vi "PH_Beamline_Chief.panel.vi"(0 "object ref":refnum<vi>, 5 "error in (no error)":errorcluster) -> (19 "error out":errorcluster)   [LabVIEW 2014, in "PH_Beamline_Chief.lvlib"]
doc: "By this VI a hardware switch can be monitored and switched. \n\nThe indicators \"FALSE\", \"TRUE\" and \"SWITCH STATE\" show the value of the Beckhoff-Tag: blue indicates bad tag status reference problems, darkgreen false and lightgreen true. If everything is working fine, \"FALSE\" and \"SWITCH STATE\" should show the same value, while \"TRUE\" has the opposite value. The caption of the sensors for \"FALSE\" and \"TRUE\" are taken out of the database. In case of only one or no sensor these GUI elements are not shown at all.\n\nThe oval button switches. It should be in the same state as the \"SWITCH STATE\" indicator. \n\n\"Delete Instance\" disconnects and removes the instance from the PCS.\n\n\nLicense Agreement for this software:\n\nCopyright (C)\nGesellschaft für Schwerionenforschung, GSI\nPlanckstr. 1\n64291 Darmstadt\nGermany\n\nContact: D.Beck@gsi.de \n\nThis program is free software; you can redistribute it and/or modify it under the terms of the GNU General Public License as published by the Free Software Foundation; either version 2 of the license, or (at your option) any later version.\n\nThis program is distributed in the hope that it will be useful, but WITHOUT ANYW ARRANTY; without even the implied warranty of MERCHANTABILITY or FITNESS FOR A PARTICULAR PURPOSE. See the GNU General License for more details (http://www.gnu.org).\n\nGesellschaft für Schwerionenforschung, GSI\nPlanckstr. 1, 64291 Darmstadt, Germany\nFor all questions and ideas contact: M.Richter@gsi.de, H.Brand@gsi.de or D.Beck@gsi.de.\nLast update: 18-DEC-2002"
uses:
  PH_Beamline_Chief.lvlib
  PH_Basics/PH_Common/Picture/PH_Picture.GUI Element 48x48.ctl
  PH_Basics/PH_Common/Picture/PH_Picture.GUI Element 36x36.ctl
  PH_Basics/PH_Common/Picture/PH_Picture.GUI Element 24x36.ctl
  PH_Basics/PH_Common/Picture/PH_Picture.GUI Element.ctl
  PH_Basics/PH_Common/Picture/PH_Picture.GUI Element 36x24.ctl
  PH_Basics/PH_Common/Picture/PH_Picture.GUI Element 60x12.ctl
  PH_Basics/PH_Common/Picture/PH_Picture.GUI Element 12x60.ctl
  PH_Beamline/PH_Beamline.Operation Mode.ctl
  PH_Beamline/PH_Beamline.Switch Instances.ctl
  PH_Beamline/PH_Beamline.6P Switch Instances.ctl
  PH_Beamline/PH_Beamline.Black Box Instances.ctl
  PH_Beamline/PH_Beamline.Switch GUI Instances.ctl
  PH_Beamline/PH_Beamline.Switch+6P Instances.ctl
  PH_Beamline_Chief.Settings.ctl
  PH_Beamline/PH_Beamline.Force Sensor Instances.ctl
  PH_Basics/PH_SystemInformation/PH_SystemInformation.GUI Refs.ctl
  PH_BL-Master/PH_BL-Master.GUI Refs.ctl
  PH_Beamline/PH_Beamline.GUI Refs.ctl
  CS_Core/CSObj/CSObj.lvlib
  PH_Basics/PH_Common/PH_Common.lvlib
  PH_BL-Master/PH_BL-Master.lvlib
  PH_Basics/PH_SystemInformation/PH_SystemInformation.lvlib
  PH_Basics/PH_Class/PH_Class.lvlib
  PH_Beamline/PH_Beamline.lvlib
  CS_Core/CSSystem/CSSystemLib/CSSystemLib.lvlib
panel:
  in  "Force Sensor Instances":T1="MM1_ForceSensor"
  in  "Switch and 6P Instances":T2="BL_Position_MM5::MA_MM5_6PGUI"
  in  "Switch GUI Instances":T3="Shutter_Exp_Laserbay_Interlock"
  in  "Black Box Instances":T4="PA_CH1_BB"
  in  "6P Switch Instances":T5="COS_Sensitivity_Switch"
  in  "Switch Instances":T6="MA01_CH1"
  out "Exp.-Shutters closed":bool
  in  "Remote Desktop Connection":bool
  out "PHELIX_Beckhoff_Watchdog":bool caption="Failure Beckhoff"
  out "PHELIX_Timing_Mode":enum32{"10 Hz", "0.5 Hz", "Shot"}(radio) caption="Modeselector"
  out "Emergency Off":u32(colorbox)
  out "Igni FR: Heating off":bool
  out "Igni MA 5: Heating off":bool
  out "Igni MA 4: Heating off":bool
  out "Igni MA 3: Heating off":bool
  out "Igni MA 2: Heating off":bool
  out "Igni MA 1: Heating off":bool
  in  "Z6 Main":bool
  in  "PCS Main":bool
  in  "PCS System Indicator":bool caption="PCS"
  in  "CoG":bool
  in  "Calibrator":bool
  in  "Image Statistician":bool
  out "Shutter_Exp3":bool=TRUE
  out "Shutter_Exp2":bool=TRUE
  out "Shutter_Exp1":bool=TRUE
  out "Shutter Exp 4 (Z6)":u32(colorbox)
  out "Shutter Exp 3":u32(colorbox)
  out "Shutter Exp 2":u32(colorbox)
  out "Shutter Exp 1":u32(colorbox)
  in  "Tab Control":T7(tab)=enum."In.-Box"
  in  "\"D:\\PCS\\Remote Access\\ns.rdp\"":bool caption="OK Button"
  out "ns Frontend ok":bool caption="ok"
  out "ns_WP_RR_6PWpGUI":T8
  in  "Hop 15":bool
  out "BL ns 8":u32(colorbox)
  out "NS_Shut_PA_BB":bool=TRUE
  out "BL ns 7":u32(colorbox)
  out "BL ns 6":u32(colorbox)
  out "BL ns 5":u32(colorbox)
  out "BL ns 4":u32(colorbox)
  out "BL ns 3":u32(colorbox)
  out "BL ns 2":u32(colorbox)
  out "BL ns 1":u32(colorbox)
  out "ns_Nearfield_Ring_Exit_ImageOperator":bool=TRUE
  out "ns_Nearfield_Ring_Exit_Cam":bool=TRUE
  out "ns_Farfield_Ring_Exit_ImageOperator":bool=TRUE
  out "ns_Farfield_Ring_Exit_Cam":bool=TRUE
  out "ns_Exit_Powermeter":bool=TRUE
  in  "Hop 23":bool
  in  "\"D:\\PCS\\Remote Access\\fs.rdp\"":bool caption="OK Button"
  out "fs Frontend ok":bool caption="ok"
  out "BL fs 17":u32(colorbox)
  out "BL fs 16":u32(colorbox)
  out "YLF_WP_6PWpGUI":T9
  out "fs_WP_Exit_6PWpGUI":T8
  out "fs_OO_Spectrometer":bool=TRUE
  out "BL fs 8":u32(colorbox)
  out "BL fs 10":u32(colorbox)
  out "fs_RR_Cavity_NF2GUI":T10
  out "fs_Stretcher_6PGUI":T10
  out "BL fs 15":u32(colorbox)
  out "FS_Shut_PA_BB":bool=TRUE
  out "BL fs 14":u32(colorbox)
  in  "Hop 3":bool
  out "BL fs 13":u32(colorbox)
  out "FS_Switch_YLF_BB":T10
  out "BL fs 12":u32(colorbox)
  out "BL fs 11":u32(colorbox)
  out "BL fs 7":u32(colorbox)
  out "BL fs 5":u32(colorbox)
  out "BL fs 9":u32(colorbox)
  out "BL fs 6":u32(colorbox)
  out "BL fs 4":u32(colorbox)
  out "BL fs 3":u32(colorbox)
  out "BL fs 2":u32(colorbox)
  out "BL fs 1":u32(colorbox)
  out "fs_Nearfield_Frontend_ImageOperator":bool=TRUE
  out "fs_Nearfield_Frontend_Cam":bool=TRUE caption="fs NF Exit Cam"
  out "fs_Synchrolock_Watch":bool=TRUE
  out "uOPA ok":bool caption="ok"
  in  "\"D:\\PCS\\Remote Access\\uOPA.rdp\"":bool caption="OK Button"
  out "BL uOPA 9":u32(colorbox)
  out "uOPA_Pump_OO_Spectrometer":bool=TRUE
  out "uOPA_Pump_WP_6PWpGUI":T8
  out "BL uOPA 8":u32(colorbox)=6618880
  out "BL uOPA 7":u32(colorbox)
  out "BL uOPA 6":u32(colorbox)
  out "BL uOPA 5":u32(colorbox)
  out "BL uOPA 4":u32(colorbox)
  out "BL uOPA 3":u32(colorbox)
  out "BL uOPA 2":u32(colorbox)
  out "BL uOPA 1":u32(colorbox)
  out "BL uOPA 0":u32(colorbox)
  in  "Hop 24":bool
  out "uOPA_Regen_Cam":bool=TRUE
  out "uOPA_Pump_Powermeter":bool=TRUE
  out "PA_Input_2_Beam_6PWpGUI":T8
  out "BL PA 21":u32(colorbox)
  out "BL PA 11":u32(colorbox)
  out "PA_ML_T3_Exit_6P4QGUI":T8 caption="PA Lens"
  out "PA_SA_6P4QGUI":T10
  out "PA_CH1_BB":T11 caption="CH"
  out "BL PA 4":u32(colorbox)
  out "PA_Input_Delay_6PGUI":T10
  out "BL PA 8":u32(colorbox)
  out "BL PA 7":u32(colorbox)
  out "BL PA 6":u32(colorbox)
  out "BL PA 5":u32(colorbox)
  out "BL PA 3":u32(colorbox)
  out "PA_non_delayed_BB":bool=TRUE
  out "PA_delayed_BB":bool=TRUE
  out "PA-Backreflection-Meas":bool=TRUE
  out "PA_PC_WP_2_BB":bool=TRUE
  in  "Hop 22":bool
  in  "Hop 16":bool
  out "BL PA 20":u32(colorbox)
  out "PA_PC_WP_BB":bool=TRUE
  out "PA_PiH_VSF2_6PGUI":T8
  out "BL PA 10":u32(colorbox)
  out "PA_Shut_Input_BB":bool=TRUE
  out "PA_PiH_VSF4_6PGUI":T8
  in  "Hop 6":bool
  in  "Hop 5":bool
  in  "Hop 4":bool
  out "PA_MM_P_Input_NF2GUI":T10
  out "PA_MM_C_Input_NF2GUI":T10
  out "BL PA 0":u32(colorbox)
  out "BL PA 16":u32(colorbox)
  out "BL PA 12":u32(colorbox)
  out "BL PA 14":u32(colorbox)
  out "PA_VacuumControl::PA_VacuumControl_Telescope 2":dbl=2000.0 caption="mbar" format="%#_2e"
  out "PA_VacuumControl::PA_VacuumControl_Telescope 3":dbl=2000.0 caption="mbar" format="%#_2e"
  out "PA_VacuumControl::PA_VacuumControl_Telescope 4":dbl=2000.0 caption="mbar" format="%#_2e"
  out "PA_VacuumControl::PA_VacuumControl_Bridge":dbl=2000.0 caption="mbar" format="%#_2e"
  out "BL PA 18":u32(colorbox)
  out "BL PA 17":u32(colorbox)
  out "PA_Bypass_Out":T10
  out "PA_Bypass_In":T10
  out "BL PA 22":u32(colorbox)
  out "PA_Switch_Lab_BB":T10
  out "PA_Exit_Shut_BB":bool=TRUE
  out "BL PA 19":u32(colorbox)
  out "BL PA 15":u32(colorbox)
  out "BL PA 13":u32(colorbox)
  out "PA_Nearfield_Input_ImageOperator":bool=TRUE
  out "PA_Nearfield_Input_Cam":bool=TRUE
  out "PA_Farfield_Input_ImageOperator":bool=TRUE
  out "PA_Farfield_Input_Cam":bool=TRUE
  out "BL PA 9":u32(colorbox)
  out "BL PA 1":u32(colorbox)
  out "PA_VacuumControl::PA_VacuumControl_Telescope 1":dbl=2000.0 caption="mbar" format="%#_2e"
  out "PA_VacuumControl::PA_VacuumControl_PA global":dbl=2000.0 caption="mbar" format="%#_2e"
  out "BL PA 2":u32(colorbox)
  out "PreAmp ok":bool caption="ok"
  in  "\"D:\\PCS\\Remote Access\\PA-Input.rdp\"":bool caption="OK Button"
  out "PA ED ok":bool caption="ok"
  in  "\"D:\\PCS\\Remote Access\\PA-Exit.rdp\"":bool caption="OK Button"
  out "PA_ED_FILT1_BB":bool=TRUE
  in  "Hop 7":bool
  out "PA_Exit_Powermeter":bool=TRUE
  out "BL PA ED 2":u32(colorbox)
  out "PA_WP_Exit_6PWpGUI":T9
  out "PA_Farfield_Exit_ImageOperator":bool=TRUE
  out "PA_Farfield_Exit_Cam":bool=TRUE caption="PA FF Exit Cam"
  out "PA_Nearfield_Exit_ImageOperator":bool=TRUE
  out "PA_Nearfield_Exit_Cam":bool=TRUE caption="PA NF Exit Cam"
  out "PA_ED_FILT2_BB":T9 caption="Filt 2"
  out "BL PA ED 1":u32(colorbox)
  out "MA_ML_In_6P4QGUI":T8 caption="PA Lens"
  out "PA_Bridge_CH_Input_MA_BB":T11 caption="CH"
  out "BL MA-IB 9":u32(colorbox)
  out "BL MA-IB 8":u32(colorbox)
  out "BL MA-IB 14":u32(colorbox)
  out "BL MA-IB 12":u32(colorbox)
  out "BL MA-IB 13":u32(colorbox)
  out "MA_Nearfield_PiH_out_ImageOperator":bool=TRUE
  out "MA_Nearfield_PiH_out_Cam":bool=TRUE
  out "MA_InB_IM_Out_Switch":T10
  out "MA_InB_DP_Out_Switch":bool=TRUE
  out "MA_InB_DP_In_Switch":bool=TRUE
  out "BL MA-IB 11":u32(colorbox)
  out "BL MA-IB 10":u32(colorbox)
  out "MA_InB_IM_In_Switch":T10
  out "BL MA-IB 7":u32(colorbox)
  out "BL MA-IB 6":u32(colorbox)
  out "BL MA-IB 5":u32(colorbox)
  out "MA_Diffusor_Inject_In_BB":bool=TRUE
  out "BL MA-IB 4":u32(colorbox)
  out "BL MA-IB 3":u32(colorbox)
  out "BL MA-IB 2":u32(colorbox)
  out "BL MA-IB 1":u32(colorbox)
  out "PA_C_MA_6PGUI":T10
  out "MA_Inject_In_ImageOperator":bool=TRUE
  out "MA_Inject_In_Cam":bool=TRUE
  out "MA_Inject_P_6PGUI":T10
  in  "Hop 2":bool
  in  "Hop 1":bool
  out "MA_Nearfield_PiH_in_ImageOperator":bool=TRUE
  out "MA_Nearfield_PiH_in_Cam":bool=TRUE
  out "MA_Inject_C_NF2GUI":T10
  out "MA_IB_Ready":bool
  out "PA_MA_Bridge_Input_Cam":bool=TRUE
  in  "\"D:\\PCS\\Remote Access\\MA.rdp\"":bool caption="OK Button"
  out "In.-Box ok":bool caption="ok"
  out "MM1_ForceSensor":bool
  in  "\"D:\\PCS\\Remote Access\\MA.rdp\" 2":bool caption="OK Button"
  out "FR+MT_Flowbox_off":bool caption="Flowboxes FR + MT off"
  out "MainAmp_Flowbox_off":bool caption="Flowboxes MA off"
  out "MainAmp ok":bool caption="ok"
  out "MA01_CH1":T11 caption="CH"
  out "MA01_CH2":T11 caption="CH"
  out "MA01_CH4":T11 caption="CH"
  out "MA01_CH3":T11 caption="CH"
  out "BL MA 3":u32(colorbox)
  out "BL MA 9":u32(colorbox)
  in  "Hop 11":bool
  out "BL MA 8":u32(colorbox)
  out "MA_Shut_AlignCam_BB":bool=TRUE
  out "MA01_O2_Beamline_MM3":dbl=99.0 caption="%O2" format="%#_2f"
  out "MA01_O2_Beamline_MM1":dbl=99.0 caption="%O2" format="%#_2f"
  in  "Hop 9":bool
  in  "Hop 8":bool
  out "MA_Alignment_ImageOperator":bool=TRUE
  out "MA_Alignment_Cam":bool=TRUE
  out "BL MA 7":u32(colorbox)
  out "BL MA 2":u32(colorbox)
  out "MA_VacuumControl::MA_VacuumControl_MA Telescope Prepressure":dbl=2000.0 caption="mbar" format="%#_6e"
  out "BL MA 6":u32(colorbox)
  out "BL MA 5":u32(colorbox)
  out "BL MA 4":u32(colorbox)
  out "BL MA 1":u32(colorbox)
  out "MA_VacuumControl::MA_VacuumControl_MA Telescope":dbl=2000.0 caption="mbar" format="%#_6e"
  out "MA_MM3_6PGUI":T12
  out "MA_MM1_6P4QGUI":T12
  out "MA_MM4_6PGUI":T12
  out "MA_MM2_6PGUI":T12
  out "MA_MM1_Bend_6P4QGUI":T12
  in  "\"D:\\PCS\\Remote Access\\MAS.rdp\"":bool caption="OK Button"
  out "MAS ok":bool caption="ok"
  out "MAS_SHS_Cam":bool=TRUE
  out "MAS_FF_HamamatsuCam":bool=TRUE
  out "MAS_Attenuator_3_BB":T9
  out "MAS_Attenuator_2_BB":T9
  out "MAS_OO_Spectrometer":bool=TRUE
  out "MAS_Discrete_Spectro_Rev6PGUI":T8
  out "BL MAS 3":u32(colorbox)
  in  "Hop 10":bool
  out "MAS_Beam_Fine_Attenuator_6PWpGUI":T8
  out "MAS_Farfield_High_Res_ImageOperator":bool=TRUE
  out "MAS_Farfield_High_Res_Cam":bool=TRUE
  out "BL MAS 5":u32(colorbox)
  out "MAS_Nearfield_ImageOperator":bool=TRUE
  out "MAS_Nearfield_Cam":bool=TRUE
  out "BL MAS 4":u32(colorbox)
  out "MAS_Attenuator_1_BB":bool=TRUE
  out "BL MAS 2":u32(colorbox)
  out "MAS_Powermeter":bool=TRUE
  out "BL MAS 1":u32(colorbox)
  out "Booster ok":bool caption="ok"
  out "BL Boo 5":u32(colorbox)
  in  "Hop 17":bool
  out "MA_MM8_6PGUI":T10
  in  "Hop 13":bool
  out "BL Boo 4":u32(colorbox)
  in  "Hop 12":bool
  out "BL Boo 3":u32(colorbox)
  out "BL Boo 2":u32(colorbox)
  out "BL Boo 1":u32(colorbox)
  out "BL_Position_MM5::MA_MM5_6PGUI":T10
  out "Calorimeter_Switch":bool=TRUE
  in  "\"D:\\PCS\\Remote Access\\COS.rdp\"":bool caption="OK Button"
  out "Compressor ok":bool caption="ok"
  out "Compressor_Grating_1_6PGUI":T13
  out "Compressor_Grating_2_6PGUI":T13
  out "COS_Filt1_BB":bool=TRUE
  out "COS-SSAC":bool=TRUE
  out "COS_SSAC_Cam":bool=TRUE
  out "COS_WP_6PWpGUI":T8
  out "COS_Filt2_BB":T8 caption="Filt 2"
  out "BL Compressor 8":u32(colorbox)
  out "COS_Sensitivity_Switch":bool=TRUE
  out "COS_NF_Cam":bool=TRUE
  out "COS_FF_Cam":bool=TRUE
  out "Compressor_VacuumControl::Compressor_VacuumControl_Compressor Pre":dbl=2000.0 caption="mbar" format="%#_6e"
  out "Compressor_VacuumControl::Compressor_VacuumControl_Compressor":dbl=2000.0 caption="mbar" format="%#_6e"
  out "BL Compressor 5":u32(colorbox)
  out "BL Compressor 6":u32(colorbox)
  out "BL Compressor 7":u32(colorbox)
  out "Compressor_LM_6PGUI":T10
  out "BL Compressor 4":u32(colorbox)
  out "BL Compressor 2":u32(colorbox)
  out "BL Compressor":u32(colorbox)
  out "Compressor_Grating_1_Tip+Tilt_6PGUI":T10
  out "Compressor_Grating_2_Tip+Tilt_6PGUI":T10
  in  "Hop 19":bool
  in  "Hop 20":bool
  out "BL Compressor 3":u32(colorbox)
  out "Vacuum no shotcond Comp LB":bool caption="Vacuum is no shot condition!"
  in  "\"D:\\PCS\\Remote Access\\Experiment.rdp\"":bool caption="OK Button"
  out "Intensity LB below Limit":bool caption="I < 1E18W/cm²"
  out "HV room locked?":i32(ring) caption="Enabling State" items=["no info", "HV room open", "HV room locked"]
  out "Shutter_Exp_Laserbay_Interlock":bool caption="request Light"
  out "Laserbay evacuated?":i32(ring) caption="Enabling State" items=["no info", "LB not evacuated", "LB evacuated"]
  out "Exp: Shotmode":T14 caption="Enabling State" items=["no info", "no Shotmode", "Shotmode"]
  out "Experiment LB ok":bool caption="ok"
  out "BL Exp LB 8":u32(colorbox)
  out "BL Exp LB 7":u32(colorbox)
  out "BL Exp LB 6":u32(colorbox)
  out "Windowshutter_TB3_Watch":bool=TRUE
  out "Experiment_VacuumControl::Experiment_VacuumControl_Experiment Pirani":dbl=2000.0 caption="mbar" format="%#_6e"
  out "Experiment_VacuumControl::Experiment_VacuumControl_Experiment":dbl=2000.0 caption="mbar" format="%#_6e"
  out "Windowshutter_TB2_Watch":bool=TRUE
  out "BL Exp LB 5":u32(colorbox)
  out "BL Exp LB 4":u32(colorbox)
  out "Shutter_Exp_Laserbay":bool=TRUE
  out "Experiment_Targetmanipulator_6PGUI":T10
  out "Experiment_Targetmanipulator_TRANS_6PGUI":T15
  out "Experiment_Targetmanipulator_TURN_6PGUI":T10
  out "Compressor_Turnbox_2_Trans_6PGUI":T13
  in  "Hop 18":bool
  out "BL Exp LB 3":u32(colorbox)
  out "BL Exp LB":u32(colorbox)
  out "Compressor_Turnbox_2_6PGUI":T10
  out "BL Exp LB 2":u32(colorbox)
  out "Compressor_Turnbox_1_Trans_6PGUI":T13
  out "Compressor_Turnbox_1_6PGUI":T10
  out "MA_VacuumControl::MA_VacuumControl_Z6 Telescope BL Prepressure":dbl=2000.0 caption="mbar" format="%#_2e"
  out "Shutter_Exp4":bool=TRUE
  out "BL-Z6-CH9":T11 caption="CH"
  in  "Z6 Beamline":bool
  out "BL MT 4":u32(colorbox)
  out "MA_VacuumControl::MA_VacuumControl_Z6 Telescope BL":dbl=2000.0 caption="mbar" format="%#_2e"
  in  "Hop 14":bool
  out "BL MT 3":u32(colorbox)
  out "BL MT 2":u32(colorbox)
  out "BL MT 1":u32(colorbox)
  out "MA_MM9_6PGUI":T10
  out "BL-Z6-Beamdump":bool=TRUE
  out "Mirrortower ok":bool caption="ok"
  out "Laserlab ok":bool caption="ok"
  in  "\"D:\\PCS\\Remote Access\\Laserlabor.rdp\"":bool caption="OK Button"
  out "LL_Comp_FF_Cam":bool=TRUE
  out "LL-SSAC":bool=TRUE
  out "LL_SSAC_Cam":bool=TRUE
  out "BL LL 14":u32(colorbox)
  out "LL_Shut_Comp_Output_BB":bool=TRUE
  out "LL_Comp_Input_Cam":bool=TRUE caption="fs NF Exit Cam"
  out "BL LL 13":u32(colorbox)
  out "BL LL 12":u32(colorbox)
  out "LL_Comp_Length_6PGUI":T15
  out "LL_Comp_Grating_Rot_6PGUI":T10
  out "LL_Shut_Comp_FF_BB":bool=TRUE
  out "BL LL 11":u32(colorbox)
  out "LL_Shut_Comp_Input_BB":bool=TRUE
  out "BL LL 10":u32(colorbox)
  out "BL LL 9":u32(colorbox)
  out "LL_Comp_P_6PGUI":T10
  out "BL LL 8":u32(colorbox)
  out "LL_Comp_C_6PGUI":T10
  out "BL LL 7":u32(colorbox)
  out "BL LL 6":u32(colorbox)
  out "PA_LL_CH_Output_BB":bool=TRUE
  out "PA_LL_Output_Cam":bool=TRUE caption="PA NF Exit Cam"
  out "Intensity LL below Limit":bool caption="I < 1E18W/cm²"
  out "BL LL 5":u32(colorbox)
  out "PA_LL_CH_Input_BB":bool=TRUE
  out "BL LL 4":u32(colorbox)
  out "BL LL 3":u32(colorbox)
  out "BL LL 2":u32(colorbox)
  out "PA_LL_P_6PGUI":T10
  out "PA_LL_C_6PGUI":T10
  out "Shutter_Laserlab_Interlock":bool caption="request Light"
  out "BL LL 1":u32(colorbox)
  out "BL LL 0":u32(colorbox)
  in  "Hop 21":bool
  out "Shutter_Laserlab":bool=TRUE
  out "Laserlab evacuated?":i32(ring) caption="Enabling State" items=["no info", "LL not evacuated", "LL evacuated"]
  out "LL: Shotmode":T14 caption="Enabling State" items=["no info", "no Shotmode", "Shotmode"]
  out "PA_LL_Input_Cam":bool=TRUE caption="PA FF Exit Cam"
  in  "Settings":T16
  out "Ready for Shot":bool
  out "MainAmp enabled":u32(colorbox)
  out "Laser enabled":u32(colorbox)
  out "PreAmp enabled":u32(colorbox)
  in  "Minimize":bool
  in  "Delete":bool
  # "PCS"
  # "3.40"
  # "Stretcher"
  # "PL8000"
  # "PL9000"
  # "YLF"
  # "MIRA"
  # "Lin Regen"
  # "Ring  Regen"
  # "Verdi"
  # "Fiber Amplifier"
  # "Regen"
  # "19-2"
  # "19-1"
  # "45"
  # "2"
  # "1"
  # "MM3"
  # "1"
  # "2"
  # "3"
  # "SHS"
  # "H"
  # "2"
  # "1"
  # "Laserbay          Laserlab"
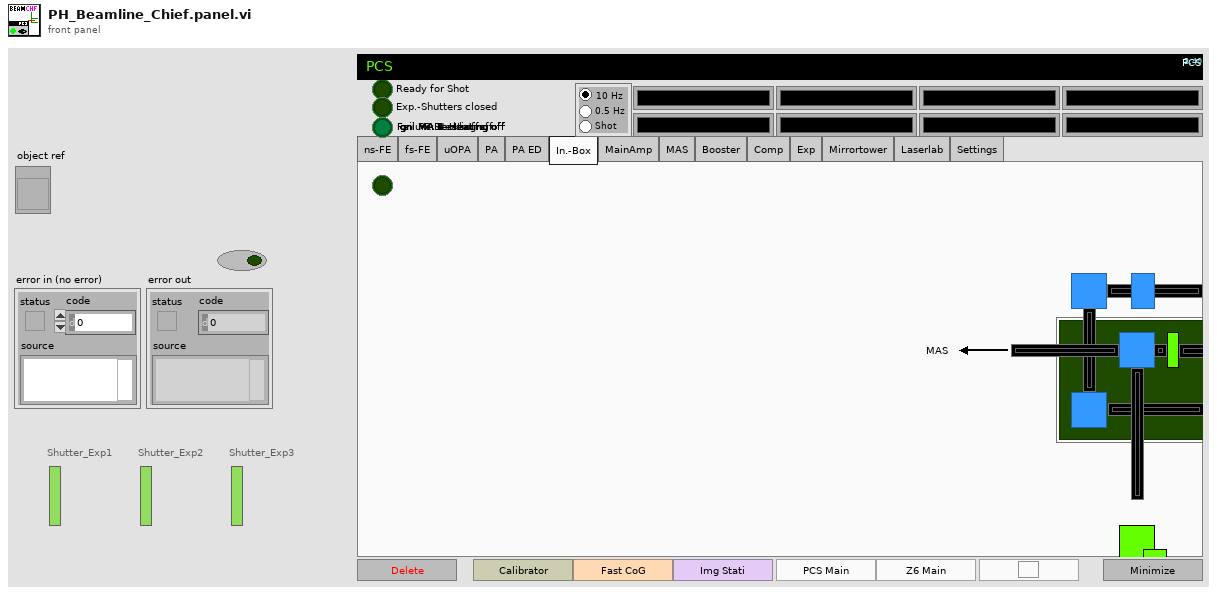
[diagram p1: front panel]
types:
  T1 = typedef "PH_Beamline.lvlib/PH_Beamline.Force Sensor Instances.ctl" = string
  T2 = typedef "PH_Beamline.lvlib/PH_Beamline.Switch+6P Instances.ctl" = string
  T3 = typedef "PH_Beamline.lvlib/PH_Beamline.Switch GUI Instances.ctl" = string
  T4 = typedef "PH_Beamline.lvlib/PH_Beamline.Black Box Instances.ctl" = string
  T5 = typedef "PH_Beamline.lvlib/PH_Beamline.6P Switch Instances.ctl" = string
  T6 = typedef "PH_Beamline.lvlib/PH_Beamline.Switch Instances.ctl" = string
  T7 = enum32{"ns-FE", "fs-FE", "uOPA", "PA", "PA ED", "In.-Box", "MainAmp", "MAS", "Booster", "Comp", "Exp", "Mirrortower", "Laserlab", "Settings"}
  T8 = typedef "PH_Common.lvlib/PH_Picture.GUI Element 24x36.ctl" = picture
  T9 = typedef "PH_Common.lvlib/PH_Picture.GUI Element 36x24.ctl" = picture
  T10 = typedef "PH_Common.lvlib/PH_Picture.GUI Element 36x36.ctl" = picture
  T11 = typedef "PH_Common.lvlib/PH_Picture.GUI Element.ctl" = picture
  T12 = typedef "PH_Common.lvlib/PH_Picture.GUI Element 48x48.ctl" = picture
  T13 = typedef "PH_Common.lvlib/PH_Picture.GUI Element 60x12.ctl" = picture
  T14 = typedef "PH_Beamline.lvlib/PH_Beamline.Operation Mode.ctl" = i32
  T15 = typedef "PH_Common.lvlib/PH_Picture.GUI Element 12x60.ctl" = picture
  T16 = typedef "PH_Beamline_Chief.lvlib/PH_Beamline_Chief.Settings.ctl" = cluster{"PA Doublepass Mode":bool, "Compressor Vaccuum LB not relevant":bool, "Windowshutter TB2 not relevant":bool, "Windowshutter TB3 not relevant":bool}
  T17 = typedef "PH_Beamline.lvlib/PH_Beamline.GUI Refs.ctl" = cluster{"Vision on this Node?":bool, "Vision Knobs":refnum<vi>[], "GUI Refs":cluster{"PA ok":refnum<vi>, "MA ok":refnum<vi>, "fs FE ok":refnum<vi>, "ns FE ok":refnum<vi>, "PA ED ok":refnum<vi>, "MAS ok":refnum<vi>, "Booster ok":refnum<vi>, "Mirrortower ok":refnum<vi>, "In.-Box ok":refnum<vi>, "Compressor ok":refnum<vi>, "Experiment LB ok":refnum<vi>, "Experiment LL ok":refnum<vi>, "PHELIX_Beckhoff_Watchdog":refnum<vi>, "Shutters closed":refnum<vi>, "uOPA ok":refnum<vi>, "Vacuum no shotcond Comp LB":refnum<vi>}, "PP Igni Heating GUI Refs":refnum<vi>[], "Refs BL PA":cluster{"undelayed Line before Shutter":refnum<vi>[], "undelayed Line after Shutter":refnum<vi>[], "before Bypass":refnum<vi>[], "delayed Line before Shutter":refnum<vi>[], "delayed Line after Shutter":refnum<vi>[], "before Shutter Input":refnum<vi>[], "after Shutter Input":refnum<vi>[], "Bypass":refnum<vi>[], "before Shutter Exit":refnum<vi>[], "after Shutter Exit":refnum<vi>[], "to MA":refnum<vi>[], "to Lab":refnum<vi>[]}, "Refs BL MA":refnum<vi>[], "Refs BL MA-IB":refnum<vi>[], "Refs BL fs":refnum<vi>[], "Refs BL PA ED":refnum<vi>[], "Refs BL MAS":refnum<vi>[], "Refs BL Boo":refnum<vi>[], "Refs BL ns":refnum<vi>[], "Refs BL Mirrortower":refnum<vi>[], "Refs BL Compressor":refnum<vi>[], "Refs BL Exp LB":refnum<vi>[], "Refs BL LL":refnum<vi>[], "Refs BL uOPA":refnum<vi>[], "Ref Op Mode Exp LB":refnum<vi>, "Ref Laserbay evacuated":refnum<vi>, "Ref Op Mode Exp LL":refnum<vi>, "Ref Laserlab evacuated":refnum<vi>, "Ref HV room locked":refnum<vi>, "Ref Bridge LB":refnum<vi>, "Ref Bridge LL":refnum<vi>}
  T18 = typedef "PH_BL-Master.lvlib/PH_BL-Master.GUI Refs.ctl" = cluster{"Vac GUI Refs":refnum<vi>[], "O2 GUI Refs":refnum<vi>[], "Ready for Shot":refnum<vi>, "Boolean Condition Service Subscriber GUI Refs":refnum<vi>[], "Vision ID on same Node":string, "Picture Condition Service Subscriber GUI Refs":refnum<vi>[], "6P 4Q GUI Refs":refnum<vi>[], "Ref Switch GUI Instances":refnum<vi>, "Ref 6P Switch Instances":refnum<vi>, "Ref BB Instances":refnum<vi>, "Ref Switch Instances":refnum<vi>, "Ref Switch and 6P State Instances":refnum<vi>, "Boolean Status Service Subscriber GUI Refs":refnum<vi>[], "Picture Status Service Subscriber GUI Refs":refnum<vi>[], "Force Sensor Instances":refnum<vi>, "GUI Ref Delete":refnum<vi>}
  T19 = typedef "PH_SystemInformation.lvlib/PH_SystemInformation.GUI Refs.ctl" = cluster{"Laser":refnum<vi>, "PreAmp":refnum<vi>, "MainAmp":refnum<vi>, "Emergency Off":refnum<vi>, "Exp 1":refnum<vi>, "Exp 2":refnum<vi>, "Exp 3":refnum<vi>, "Exp 4":refnum<vi>, "Timing Mode GUI Ref":refnum<vi>}
  T20 = cluster{"undelayed Line before Shutter":refnum<vi>[], "undelayed Line after Shutter":refnum<vi>[], "before Bypass":refnum<vi>[], "delayed Line before Shutter":refnum<vi>[], "delayed Line after Shutter":refnum<vi>[], "before Shutter Input":refnum<vi>[], "after Shutter Input":refnum<vi>[], "Bypass":refnum<vi>[], "before Shutter Exit":refnum<vi>[], "after Shutter Exit":refnum<vi>[], "to MA":refnum<vi>[], "to Lab":refnum<vi>[]}
  T21 = enum16{"PCS", "Laser", "Vision", "PP", "Special", "Beckhoff"}
  T22 = enum16{"None", "PCS Main", "Z6 Main", "PCS Beamline", "Z6 Beamline", "Image Statistician", "Powermeter Statistician", "SHS Anal Statistician", "Image Center of Gravity", "Image Calibrator", "SHS Analysis Calibrator", "Cam List", "Powermeterlist", "6P List", "BB List", "Switch List", "Sequence Watch"}
  T23 = typedef "PH_BL-Master.lvlib/PH_BL-Master.i attribute.ctl" = cluster{"Remote controlled":bool, "Boolean Condition Service Subscriber":refnum<vi>[], "Picture Condition Service Subscriber":refnum<vi>[], "R2S":cluster{"GUI Ref":refnum<vi>, "State":bool}, "Vacua":cluster{"GUI Ref":refnum<vi>, "Limit":dbl, "Curr Value":dbl, "in range":bool}[], "O2 Inspection":cluster{"GUI Ref":refnum<vi>, "Concentration":dbl, "State":T24}[], "Boolean Status Service Subscriber":cluster{"GUI Ref":refnum<vi>, "Status":T24, "no Link?":bool, "Status Subscriber Class":T25}[], "Picture Status Service Subscriber":cluster{"GUI Ref":refnum<vi>, "Status":T24, "no Link?":bool, "Status Subscriber Class":T25}[], "6P 4Q Service Subscriber":cluster{"GUI Ref":refnum<vi>, "Selector":T26, "no Link?":bool}[], "Index of latest 6P 4Q changing Instance":i32, "Index of latest Picture Status changing Instance":i32, "Index of latest Boolean Status changing Instance":i32, "Vision ID on same Node":string, "Start Phase over?":bool, "GUI Ref Delete":refnum<vi>}
  T24 = typedef "PH_StatusHandler.lvlib/PH_StatusHandler.Status.ctl" = i16
  T25 = typedef "PH_BL-Master.lvlib/PH_BL-Master.Status Subscriber Class.ctl" = enum16{"unknown", "Switch", "BB", "6P Switch", "Switch GUI", "Switch and 6P State", "Force Sensor"}
  T26 = typedef "PH_4_Pos_Selector.lvlib/PH_4_Pos_Selector.Position Selector.ctl" = u16
  T27 = typedef "PH_Beamline_Chief.lvlib/PH_Beamline_Chief.i attribute.ctl" = cluster{"BL Service IDs":cluster{"YLF_BL_Status":i32, "fs_BL_Status":i32, "fs_YLF_BL_Status":i32, "ns_BL_Status":i32, "PA_Input_BL_Status":i32, "PA_UnDelay_BL_Status":i32, "PA_Delay_BL_Status":i32, "PA_BL_Status":i32, "PA_Bypass_BL_Status":i32, "PA_Exit_BL_Status":i32, "PA_LL_BL_Status":i32, "LL_BL_Status":i32, "PA_MA_BL_Status":i32, "MA_Exit_BL_Status":i32, "MA_Z6_BL_Status":i32, "Z6_BL_Status":i32, "MA_LB_BL_Status":i32, "LB_TB2_BL_Status":i32, "PA_before_Bypass_BL_Status":i32, "LB_TB3_BL_Status":i32}, "R2S Service ID":i32, "Settings":cluster{"Wanted":T16, "GUI Ref":refnum<vi>, "Service ID":i32}}
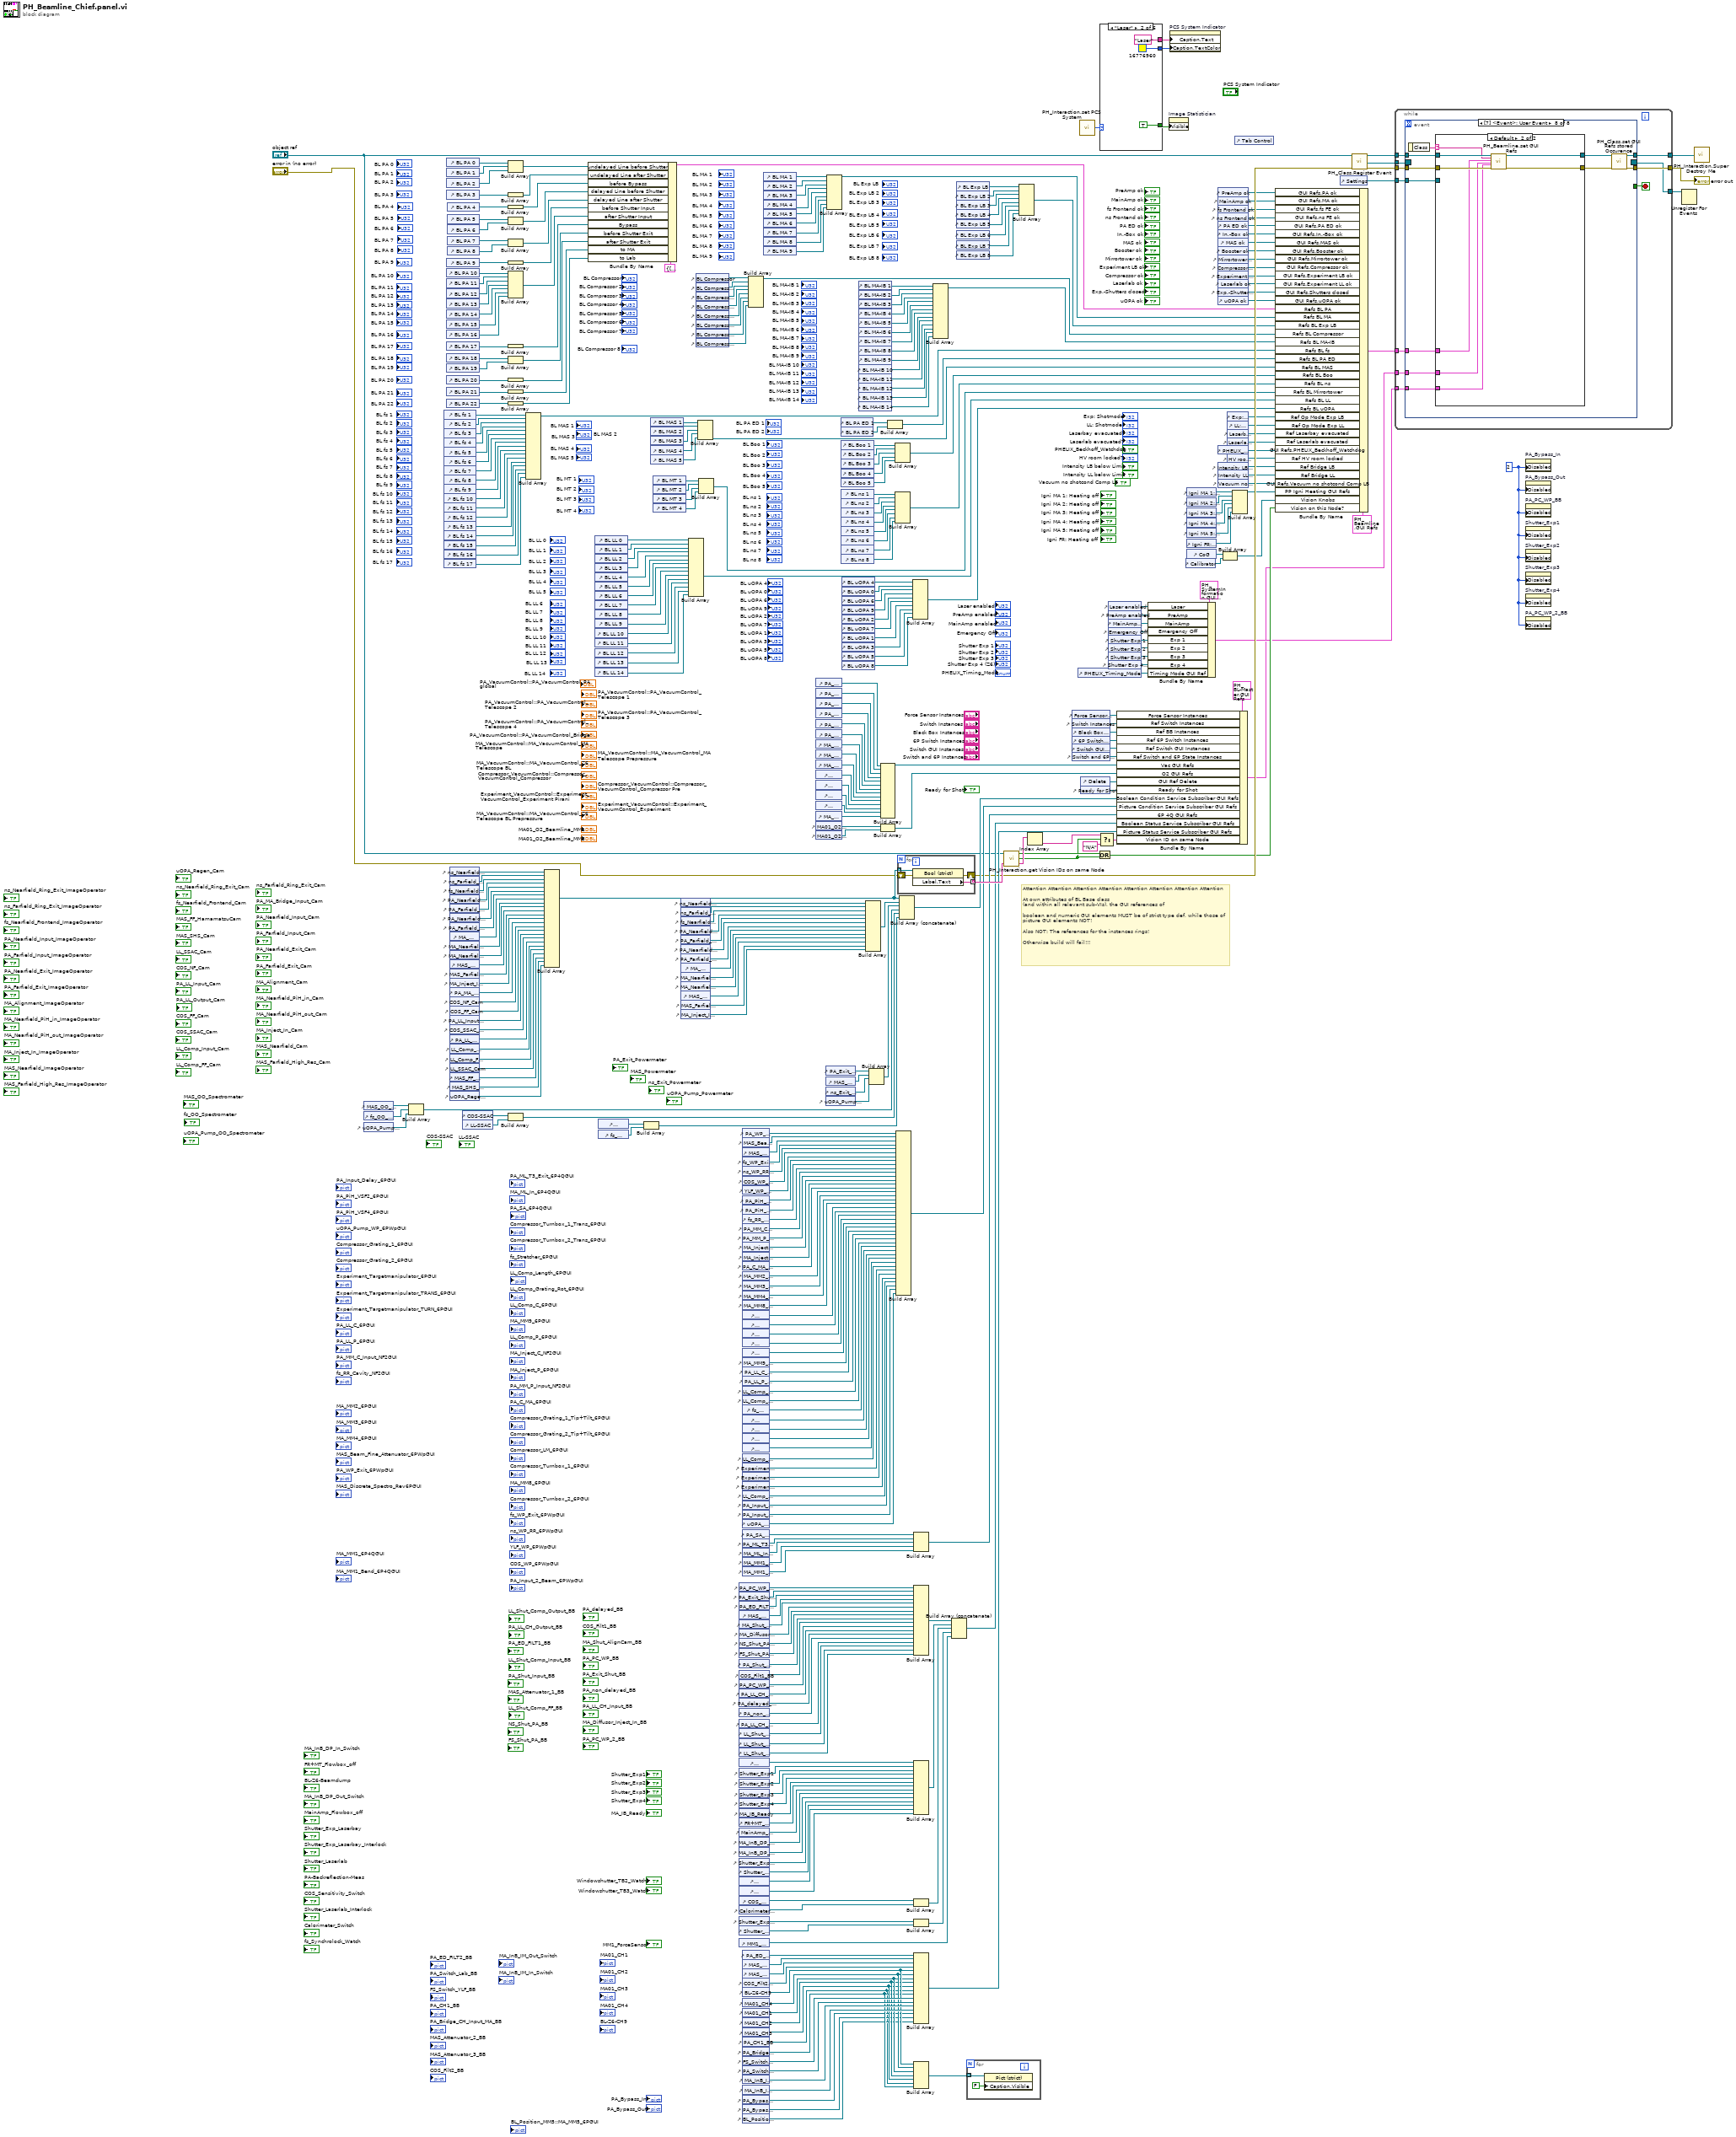
[diagram p0: block diagram]
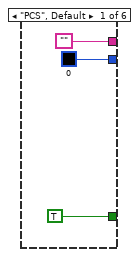
[diagram p2: hidden frame]
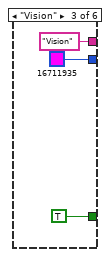
[diagram p3: hidden frame]
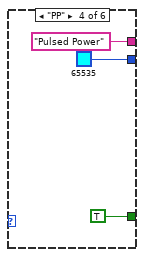
[diagram p4: hidden frame]
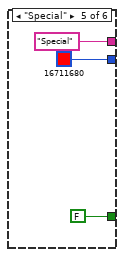
[diagram p5: hidden frame]
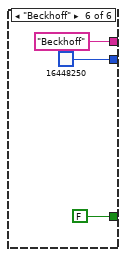
[diagram p6: hidden frame]
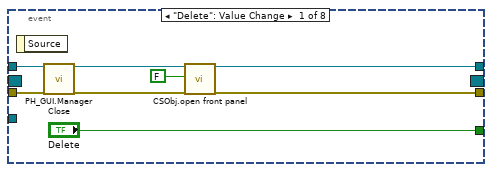
[diagram p7: hidden frame]
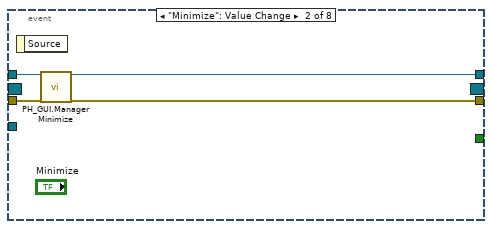
[diagram p8: hidden frame]
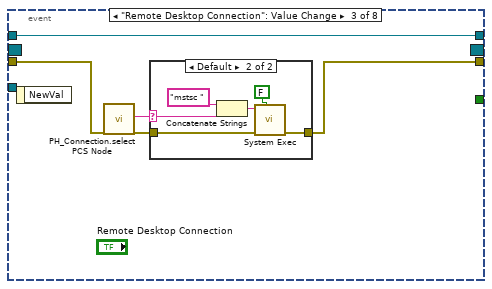
[diagram p9: hidden frame]
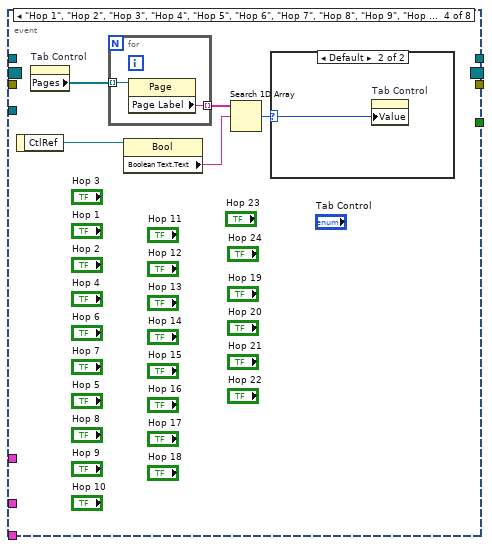
[diagram p11: hidden frame]
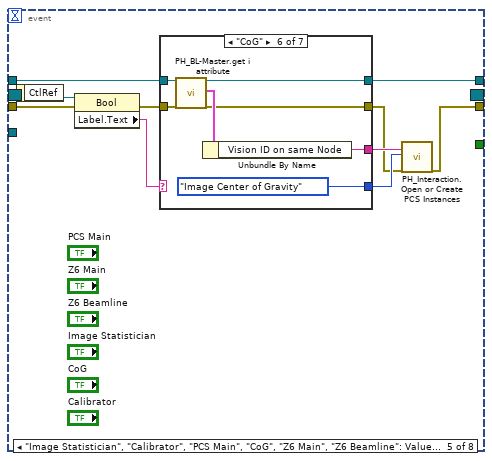
[diagram p13: hidden frame]
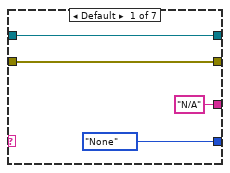
[diagram p14: hidden frame]
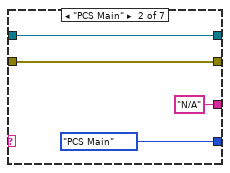
[diagram p15: hidden frame]
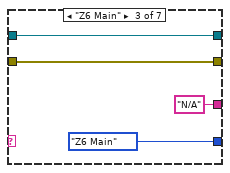
[diagram p16: hidden frame]
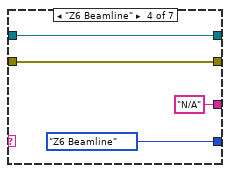
[diagram p17: hidden frame]
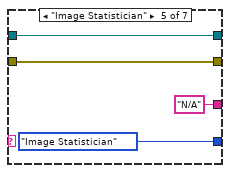
[diagram p18: hidden frame]
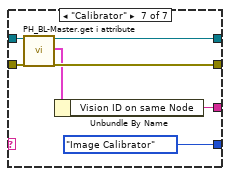
[diagram p19: hidden frame]
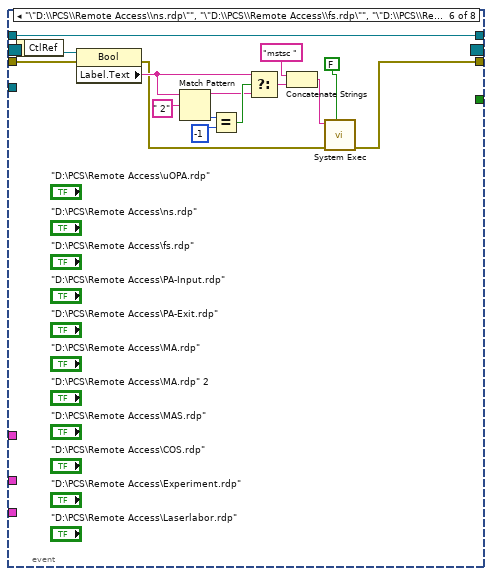
[diagram p20: hidden frame]
diagram:
  w253 = u8 2 ("Disabled")
  # "Attention Attention Attention Attention Attention Attention Attention Attention\n\nAt own attributes of BL Base class \n(and within all relevant sub-VIs), the GUI references of\n\nboolean and numeric GUI elements MUST be of strict type def, while those of\npicture GUI elements NOT!\n\nAlso NOT: The references for the instances rings!\n\nOtherwise build will fail!!!"
  n1 = control-ref of="MAS_OO_Spectrometer"() -> (w265:refnum<vi>)
  n2 = control-ref of="fs_OO_Spectrometer"() -> (w264:refnum<vi>)
  n3 = control-ref of="uOPA_Pump_OO_Spectrometer"() -> (w78:refnum<vi>)
  n4 = Build Array(w265, w264, w78) -> (w114:refnum<vi>[])
  n5 = control-ref of="BL fs 1"() -> (w375:refnum<vi>)
  n6 = control-ref of="BL fs 2"() -> (w374:refnum<vi>)
  n7 = control-ref of="BL fs 3"() -> (w373:refnum<vi>)
  n8 = control-ref of="BL fs 4"() -> (w372:refnum<vi>)
  n9 = control-ref of="BL fs 5"() -> (w371:refnum<vi>)
  n10 = control-ref of="BL fs 6"() -> (w370:refnum<vi>)
  n11 = control-ref of="BL fs 7"() -> (w369:refnum<vi>)
  n12 = control-ref of="BL fs 8"() -> (w368:refnum<vi>)
  n13 = control-ref of="BL fs 9"() -> (w367:refnum<vi>)
  n14 = control-ref of="BL fs 10"() -> (w366:refnum<vi>)
  n15 = control-ref of="BL fs 11"() -> (w365:refnum<vi>)
  n16 = control-ref of="BL fs 12"() -> (w364:refnum<vi>)
  n17 = control-ref of="BL fs 13"() -> (w363:refnum<vi>)
  n18 = control-ref of="BL fs 14"() -> (w317:refnum<vi>)
  n19 = control-ref of="BL fs 15"() -> (w277:refnum<vi>)
  n20 = control-ref of="BL fs 16"() -> (w276:refnum<vi>)
  n21 = control-ref of="BL fs 17"() -> (w275:refnum<vi>)
  n22 = control-ref of="BL PA 0"() -> (w243:refnum<vi>)
  n23 = control-ref of="BL PA 1"() -> (w242:refnum<vi>)
  n24 = control-ref of="BL PA 2"() -> (w241:refnum<vi>)
  n25 = control-ref of="BL PA 3"() -> (w239:refnum<vi>)
  n26 = control-ref of="BL PA 9"() -> (w229:refnum<vi>)
  n27 = control-ref of="BL PA 10"() -> (w227:refnum<vi>)
  n28 = control-ref of="BL PA 11"() -> (w226:refnum<vi>)
  n29 = control-ref of="BL PA 12"() -> (w225:refnum<vi>)
  n30 = control-ref of="BL PA 13"() -> (w224:refnum<vi>)
  n31 = control-ref of="BL PA 14"() -> (w223:refnum<vi>)
  n32 = control-ref of="BL PA 15"() -> (w222:refnum<vi>)
  n33 = control-ref of="BL PA 16"() -> (w221:refnum<vi>)
  n34 = control-ref of="BL PA 17"() -> (w219:refnum<vi>)
  n35 = control-ref of="BL PA 18"() -> (w217:refnum<vi>)
  n36 = control-ref of="BL PA 19"() -> (w216:refnum<vi>)
  n37 = control-ref of="BL PA 20"() -> (w214:refnum<vi>)
  n38 = control-ref of="BL PA 21"() -> (w213:refnum<vi>)
  n39 = control-ref of="BL PA 22"() -> (w212:refnum<vi>)
  n40 = control-ref of="BL PA 4"() -> (w237:refnum<vi>)
  n41 = control-ref of="BL PA 5"() -> (w235:refnum<vi>)
  n42 = control-ref of="BL PA 6"() -> (w234:refnum<vi>)
  n43 = control-ref of="BL PA 7"() -> (w232:refnum<vi>)
  n44 = control-ref of="BL PA 8"() -> (w231:refnum<vi>)
  n45 = control-ref of="ns_Nearfield_Ring_Exit_Cam"() -> (w410:refnum<vi>)
  n46 = control-ref of="ns_Farfield_Ring_Exit_Cam"() -> (w409:refnum<vi>)
  n47 = control-ref of="fs_Nearfield_Frontend_Cam"() -> (w408:refnum<vi>)
  n48 = control-ref of="PA_Nearfield_Input_Cam"() -> (w407:refnum<vi>)
  n49 = control-ref of="PA_Farfield_Input_Cam"() -> (w406:refnum<vi>)
  n50 = control-ref of="PA_Nearfield_Exit_Cam"() -> (w405:refnum<vi>)
  n51 = control-ref of="PA_Farfield_Exit_Cam"() -> (w404:refnum<vi>)
  n52 = control-ref of="MA_Alignment_Cam"() -> (w403:refnum<vi>)
  n53 = control-ref of="MA_Nearfield_PiH_in_Cam"() -> (w402:refnum<vi>)
  n54 = control-ref of="MA_Nearfield_PiH_out_Cam"() -> (w401:refnum<vi>)
  n55 = control-ref of="MAS_Nearfield_Cam"() -> (w400:refnum<vi>)
  n56 = control-ref of="MAS_Farfield_High_Res_Cam"() -> (w399:refnum<vi>)
  n57 = control-ref of="MA_Inject_In_Cam"() -> (w348:refnum<vi>)
  n58 = control-ref of="PA_MA_Bridge_Input_Cam"() -> (w316:refnum<vi>)
  n59 = control-ref of="COS_NF_Cam"() -> (w282:refnum<vi>)
  n60 = control-ref of="COS_FF_Cam"() -> (w281:refnum<vi>)
  n61 = control-ref of="PA_LL_Input_Cam"() -> (w250:refnum<vi>)
  n62 = control-ref of="COS_SSAC_Cam"() -> (w206:refnum<vi>)
  n63 = control-ref of="PA_LL_Output_Cam"() -> (w146:refnum<vi>)
  n64 = control-ref of="LL_Comp_Input_Cam"() -> (w145:refnum<vi>)
  n65 = control-ref of="LL_Comp_FF_Cam"() -> (w144:refnum<vi>)
  n66 = control-ref of="LL_SSAC_Cam"() -> (w139:refnum<vi>)
  n67 = control-ref of="MAS_FF_HamamatsuCam"() -> (w91:refnum<vi>)
  n68 = control-ref of="MAS_SHS_Cam"() -> (w90:refnum<vi>)
  n69 = control-ref of="uOPA_Regen_Cam"() -> (w79:refnum<vi>)
  n70 = control-ref of="COS-SSAC"() -> (w205:refnum<vi>)
  n71 = control-ref of="LL-SSAC"() -> (w138:refnum<vi>)
  n72 = Build Array(w243, w242, w241) -> (w240:refnum<vi>[])
  n73 = Build Array(w239) -> (w238:refnum<vi>[])
  n74 = Build Array(w237) -> (w236:refnum<vi>[])
  n75 = Build Array(w235, w234) -> (w233:refnum<vi>[])
  n76 = Build Array(w232, w231) -> (w230:refnum<vi>[])
  n77 = Build Array(w229) -> (w228:refnum<vi>[])
  n78 = Build Array(w227, w226, w225, w224, w223, w222, w221) -> (w220:refnum<vi>[])
  n79 = Build Array(w219) -> (w218:refnum<vi>[])
  n80 = Build Array(w217, w216) -> (w215:refnum<vi>[])
  n81 = Build Array(w214) -> (w211:refnum<vi>[])
  n82 = Build Array(w213) -> (w210:refnum<vi>[])
  n83 = Build Array(w212) -> (w209:refnum<vi>[])
  n84 = Build Array(w205, w138) -> (w113:refnum<vi>[])
  n85 = Build Array(w375, w374, w373, w372, w371, w370, w369, w368, w367, w366, w365, w364, w363, w317, w277, w276, w275) -> (w35:refnum<vi>[])
  n86 = Build Array(w410, w409, w408, w407, w406, w405, w404, w403, w402, w401, w400, w399, w348, w316, w282, w281, w250, w206, w146, w145, w144, w139, w91, w90, w79) -> (w103:refnum<vi>[])
  n87 = Bundle By Name(cluster=T20 {"undelayed Line before Shutter"=[], "undelayed Line after Shutter"=[], "before Bypass"=[], "delayed Line before Shutter"=[], "delayed Line after Shutter"=[], "before Shutter Input"=[], "after Shutter Input"=[], "Bypass"=[], "before Shutter Exit"=[], "after Shutter Exit"=[], "to MA"=[], "to Lab"=[]} ("Refs BL PA"), "undelayed Line before Shutter"=w240, "undelayed Line after Shutter"=w238, "before Bypass"=w236, "delayed Line before Shutter"=w233, "delayed Line after Shutter"=w230, "before Shutter Input"=w228, "after Shutter Input"=w220, "Bypass"=w218, "before Shutter Exit"=w215, "after Shutter Exit"=w211, "to MA"=w210, "to Lab"=w209) -> (w40:T20)
  n88 = control-ref of="BL LL 0"() -> (w269:refnum<vi>)
  n89 = control-ref of="BL LL 1"() -> (w268:refnum<vi>)
  n90 = control-ref of="BL LL 2"() -> (w249:refnum<vi>)
  n91 = control-ref of="BL LL 3"() -> (w248:refnum<vi>)
  n92 = control-ref of="BL LL 4"() -> (w247:refnum<vi>)
  n93 = control-ref of="BL LL 5"() -> (w245:refnum<vi>)
  n94 = control-ref of="BL LL 6"() -> (w156:refnum<vi>)
  n95 = control-ref of="BL LL 7"() -> (w155:refnum<vi>)
  n96 = control-ref of="BL LL 8"() -> (w154:refnum<vi>)
  n97 = control-ref of="BL LL 9"() -> (w153:refnum<vi>)
  n98 = control-ref of="BL LL 10"() -> (w152:refnum<vi>)
  n99 = control-ref of="BL LL 11"() -> (w151:refnum<vi>)
  n100 = control-ref of="BL LL 12"() -> (w150:refnum<vi>)
  n101 = control-ref of="BL LL 13"() -> (w149:refnum<vi>)
  n102 = control-ref of="BL LL 14"() -> (w137:refnum<vi>)
  n103 = control-ref of="PA-Backreflection-Meas"() -> (w256:refnum<vi>)
  n104 = control-ref of="fs_Synchrolock_Watch"() -> (w195:refnum<vi>)
  n105 = Build Array(w256, w195) -> (w112:refnum<vi>[])
  n106 = control-ref of="BL MAS 1"() -> (w356:refnum<vi>)
  n107 = control-ref of="BL MAS 2"() -> (w355:refnum<vi>)
  n108 = control-ref of="BL MAS 3"() -> (w92:refnum<vi>)
  n109 = control-ref of="BL MAS 4"() -> (w354:refnum<vi>)
  n110 = control-ref of="BL MAS 5"() -> (w353:refnum<vi>)
  n111 = control-ref of="BL MT 1"() -> (w333:refnum<vi>)
  n112 = control-ref of="BL MT 2"() -> (w332:refnum<vi>)
  n113 = control-ref of="BL MT 3"() -> (w331:refnum<vi>)
  n114 = control-ref of="BL MT 4"() -> (w326:refnum<vi>)
  n115 = control-ref of="ns_Nearfield_Ring_Exit_ImageOperator"() -> (w398:refnum<vi>)
  n116 = control-ref of="ns_Farfield_Ring_Exit_ImageOperator"() -> (w397:refnum<vi>)
  n117 = control-ref of="fs_Nearfield_Frontend_ImageOperator"() -> (w396:refnum<vi>)
  n118 = control-ref of="PA_Nearfield_Input_ImageOperator"() -> (w395:refnum<vi>)
  n119 = control-ref of="PA_Farfield_Input_ImageOperator"() -> (w394:refnum<vi>)
  n120 = control-ref of="PA_Nearfield_Exit_ImageOperator"() -> (w393:refnum<vi>)
  n121 = control-ref of="PA_Farfield_Exit_ImageOperator"() -> (w392:refnum<vi>)
  n122 = control-ref of="MA_Alignment_ImageOperator"() -> (w391:refnum<vi>)
  n123 = control-ref of="MA_Nearfield_PiH_in_ImageOperator"() -> (w390:refnum<vi>)
  n124 = control-ref of="MA_Nearfield_PiH_out_ImageOperator"() -> (w389:refnum<vi>)
  n125 = control-ref of="MAS_Nearfield_ImageOperator"() -> (w388:refnum<vi>)
  n126 = control-ref of="MAS_Farfield_High_Res_ImageOperator"() -> (w387:refnum<vi>)
  n127 = control-ref of="MA_Inject_In_ImageOperator"() -> (w349:refnum<vi>)
  n128 = Build Array(w269, w268, w249, w248, w247, w245, w156, w155, w154, w153, w152, w151, w150, w149, w137) -> (w29:refnum<vi>[])
  n129 = control-ref of="BL Compressor"() -> (w298:refnum<vi>)
  n130 = control-ref of="BL Compressor 2"() -> (w297:refnum<vi>)
  n131 = control-ref of="BL Compressor 3"() -> (w296:refnum<vi>)
  n132 = control-ref of="BL Compressor 4"() -> (w295:refnum<vi>)
  n133 = control-ref of="BL Compressor 5"() -> (w294:refnum<vi>)
  n134 = control-ref of="BL Compressor 6"() -> (w293:refnum<vi>)
  n135 = control-ref of="BL Compressor 7"() -> (w292:refnum<vi>)
  n136 = control-ref of="BL Compressor 8"() -> (w274:refnum<vi>)
  n137 = Build Array(w356, w355, w92, w354, w353) -> (w33:refnum<vi>[])
  n138 = Build Array(w333, w332, w331, w326) -> (w30:refnum<vi>[])
  n139 = control-ref of="PA_PC_WP_BB"() -> (w377:refnum<vi>)
  n140 = control-ref of="PA_Exit_Shut_BB"() -> (w376:refnum<vi>)
  n141 = control-ref of="PA_ED_FILT1_BB"() -> (w360:refnum<vi>)
  n142 = control-ref of="MAS_Attenuator_1_BB"() -> (w359:refnum<vi>)
  n143 = control-ref of="MA_Shut_AlignCam_BB"() -> (w350:refnum<vi>)
  n144 = control-ref of="MA_Diffusor_Inject_In_BB"() -> (w190:refnum<vi>)
  n145 = control-ref of="NS_Shut_PA_BB"() -> (w322:refnum<vi>)
  n146 = control-ref of="FS_Shut_PA_BB"() -> (w319:refnum<vi>)
  n147 = control-ref of="PA_Shut_Input_BB"() -> (w318:refnum<vi>)
  n148 = control-ref of="COS_Filt1_BB"() -> (w283:refnum<vi>)
  n149 = control-ref of="PA_PC_WP_2_BB"() -> (w255:refnum<vi>)
  n150 = control-ref of="PA_LL_CH_Input_BB"() -> (w246:refnum<vi>)
  n151 = control-ref of="PA_delayed_BB"() -> (w208:refnum<vi>)
  n152 = control-ref of="PA_non_delayed_BB"() -> (w207:refnum<vi>)
  n153 = control-ref of="PA_LL_CH_Output_BB"() -> (w143:refnum<vi>)
  n154 = control-ref of="LL_Shut_Comp_Input_BB"() -> (w142:refnum<vi>)
  n155 = control-ref of="LL_Shut_Comp_FF_BB"() -> (w141:refnum<vi>)
  n156 = control-ref of="LL_Shut_Comp_Output_BB"() -> (w140:refnum<vi>)
  n157 = control-ref of="BL-Z6-Beamdump"() -> (w334:refnum<vi>)
  n158 = control-ref of="Shutter_Exp1"() -> (w330:refnum<vi>)
  n159 = control-ref of="Shutter_Exp2"() -> (w329:refnum<vi>)
  n160 = control-ref of="Shutter_Exp3"() -> (w328:refnum<vi>)
  n161 = control-ref of="Shutter_Exp4"() -> (w327:refnum<vi>)
  n162 = control-ref of="MA_IB_Ready"() -> (w325:refnum<vi>)
  n163 = control-ref of="FR+MT_Flowbox_off"() -> (w324:refnum<vi>)
  n164 = control-ref of="MainAmp_Flowbox_off"() -> (w323:refnum<vi>)
  n165 = control-ref of="MA_InB_DP_In_Switch"() -> (w300:refnum<vi>)
  n166 = control-ref of="MA_InB_DP_Out_Switch"() -> (w299:refnum<vi>)
  n167 = control-ref of="Shutter_Exp_Laserbay"() -> (w271:refnum<vi>)
  n168 = control-ref of="Shutter_Laserlab"() -> (w270:refnum<vi>)
  n169 = control-ref of="Windowshutter_TB2_Watch"() -> (w254:refnum<vi>)
  n170 = control-ref of="Windowshutter_TB3_Watch"() -> (w194:refnum<vi>)
  n171 = control-ref of="COS_Sensitivity_Switch"() -> (w280:refnum<vi>)
  n172 = control-ref of="Calorimeter_Switch"() -> (w278:refnum<vi>)
  n173 = control-ref of="Shutter_Exp_Laserbay_Interlock"() -> (w267:refnum<vi>)
  n174 = control-ref of="Shutter_Laserlab_Interlock"() -> (w266:refnum<vi>)
  n175 = control-ref of="MM1_ForceSensor"() -> (w2:refnum<vi>)
  n176 = control-ref of="PA_WP_Exit_6PWpGUI"() -> (w187:refnum<vi>)
  n177 = control-ref of="MAS_Beam_Fine_Attenuator_6PWpGUI"() -> (w186:refnum<vi>)
  n178 = control-ref of="MAS_Discrete_Spectro_6PGUI"() -> (w185:refnum<vi>)
  n179 = control-ref of="fs_WP_Exit_6PWpGUI"() -> (w184:refnum<vi>)
  n180 = control-ref of="ns_WP_RR_6PWpGUI"() -> (w183:refnum<vi>)
  n181 = control-ref of="COS_WP_6PWpGUI"() -> (w182:refnum<vi>)
  n182 = control-ref of="YLF_WP_6PWpGUI"() -> (w181:refnum<vi>)
  n183 = control-ref of="PA_PiH_VSF2_6PGUI"() -> (w180:refnum<vi>)
  n184 = control-ref of="PA_PiH_VSF4_6PGUI"() -> (w179:refnum<vi>)
  n185 = control-ref of="fs_RR_Cavity_NF2GUI"() -> (w174:refnum<vi>)
  n186 = control-ref of="PA_MM_C_Input_NF2GUI"() -> (w173:refnum<vi>)
  n187 = control-ref of="PA_MM_P_Input_NF2GUI"() -> (w172:refnum<vi>)
  n188 = control-ref of="MA_Inject_C_NF2GUI"() -> (w171:refnum<vi>)
  n189 = control-ref of="MA_Inject_P_6PGUI"() -> (w170:refnum<vi>)
  n190 = control-ref of="PA_C_MA_6PGUI"() -> (w169:refnum<vi>)
  n191 = control-ref of="MA_MM2_6PGUI"() -> (w168:refnum<vi>)
  n192 = control-ref of="MA_MM3_6PGUI"() -> (w167:refnum<vi>)
  n193 = control-ref of="MA_MM4_6PGUI"() -> (w166:refnum<vi>)
  n194 = control-ref of="MA_MM8_6PGUI"() -> (w165:refnum<vi>)
  n195 = control-ref of="Compressor_Grating_1_Tip+Tilt_6PGUI"() -> (w164:refnum<vi>)
  n196 = control-ref of="Compressor_Grating_2_Tip+Tilt_6PGUI"() -> (w163:refnum<vi>)
  n197 = control-ref of="Compressor_LM_6PGUI"() -> (w162:refnum<vi>)
  n198 = control-ref of="Compressor_Turnbox_1_6PGUI"() -> (w161:refnum<vi>)
  n199 = control-ref of="Compressor_Turnbox_2_6PGUI"() -> (w160:refnum<vi>)
  n200 = control-ref of="MA_MM9_6PGUI"() -> (w159:refnum<vi>)
  n201 = control-ref of="PA_LL_C_6PGUI"() -> (w158:refnum<vi>)
  n202 = control-ref of="PA_LL_P_6PGUI"() -> (w157:refnum<vi>)
  n203 = control-ref of="LL_Comp_C_6PGUI"() -> (w148:refnum<vi>)
  n204 = control-ref of="LL_Comp_P_6PGUI"() -> (w147:refnum<vi>)
  n205 = control-ref of="fs_Stretcher_6PGUI"() -> (w136:refnum<vi>)
  n206 = control-ref of="Compressor_Grating_1_6PGUI"() -> (w135:refnum<vi>)
  n207 = control-ref of="Compressor_Grating_2_6PGUI"() -> (w134:refnum<vi>)
  n208 = control-ref of="Compressor_Turnbox_1_Trans_6PGUI"() -> (w133:refnum<vi>)
  n209 = control-ref of="Compressor_Turnbox_2_Trans_6PGUI"() -> (w132:refnum<vi>)
  n210 = control-ref of="LL_Comp_Length_6PGUI"() -> (w131:refnum<vi>)
  n211 = control-ref of="Experiment_Targetmanipulator_TRANS_6PGUI"() -> (w130:refnum<vi>)
  n212 = control-ref of="Experiment_Targetmanipulator_6PGUI"() -> (w129:refnum<vi>)
  n213 = control-ref of="Experiment_Targetmanipulator_TURN_6PGUI"() -> (w128:refnum<vi>)
  n214 = control-ref of="LL_Comp_Grating_Rot_6PGUI"() -> (w127:refnum<vi>)
  n215 = control-ref of="PA_Input_Delay_6PGUI"() -> (w126:refnum<vi>)
  n216 = control-ref of="PA_Input_2_Beam_6PWpGUI"() -> (w97:refnum<vi>)
  n217 = control-ref of="uOPA_Pump_WP_6PWpGUI"() -> (w76:refnum<vi>)
  n218 = control-ref of="PA_SA_6P4QGUI"() -> (w107:refnum<vi>)
  n219 = control-ref of="PA_ML_T3_Exit_6P4QGUI"() -> (w106:refnum<vi>)
  n220 = control-ref of="MA_ML_In_6P4QGUI"() -> (w96:refnum<vi>)
  n221 = control-ref of="MA_MM1_6P4QGUI"() -> (w4:refnum<vi>)
  n222 = control-ref of="MA_MM1_Bend_6P4QGUI"() -> (w3:refnum<vi>)
  n223 = control-ref of="PA_ED_FILT2_BB"() -> (w189:refnum<vi>)
  n224 = control-ref of="MAS_Attenuator_2_BB"() -> (w94:refnum<vi>)
  n225 = control-ref of="MAS_Attenuator_3_BB"() -> (w93:refnum<vi>)
  n226 = control-ref of="COS_Filt2_BB"() -> (w188:refnum<vi>)
  n227 = control-ref of="BL-Z6-CH9"() -> (w124:refnum<vi>)
  n228 = control-ref of="MA01_CH4"() -> (w123:refnum<vi>)
  n229 = control-ref of="MA01_CH1"() -> (w122:refnum<vi>)
  n230 = control-ref of="MA01_CH2"() -> (w121:refnum<vi>)
  n231 = control-ref of="MA01_CH3"() -> (w120:refnum<vi>)
  n232 = control-ref of="PA_CH1_BB"() -> (w104:refnum<vi>)
  n233 = control-ref of="PA_Bridge_CH_Input_MA_BB"() -> (w119:refnum<vi>)
  n234 = control-ref of="FS_Switch_YLF_BB"() -> (w178:refnum<vi>)
  n235 = control-ref of="PA_Switch_Lab_BB"() -> (w177:refnum<vi>)
  n236 = control-ref of="MA_InB_IM_Out_Switch"() -> (w176:refnum<vi>)
  n237 = control-ref of="MA_InB_IM_In_Switch"() -> (w175:refnum<vi>)
  n238 = control-ref of="PA_Bypass_In"() -> (w118:refnum<vi>)
  n239 = control-ref of="PA_Bypass_Out"() -> (w117:refnum<vi>)
  n240 = control-ref of="BL_Position_MM5::MA_MM5_6PGUI"() -> (w105:refnum<vi>)
  n241 = Build Array(w298, w297, w296, w295, w294, w293, w292, w274) -> (w37:refnum<vi>[])
  n242 = control-ref of="BL MA 1"() -> (w418:refnum<vi>)
  n243 = control-ref of="BL MA 2"() -> (w417:refnum<vi>)
  n244 = control-ref of="BL MA 3"() -> (w416:refnum<vi>)
  n245 = control-ref of="BL MA 4"() -> (w415:refnum<vi>)
  n246 = control-ref of="BL MA 5"() -> (w411:refnum<vi>)
  n247 = control-ref of="BL MA 6"() -> (w414:refnum<vi>)
  n248 = control-ref of="BL MA 7"() -> (w413:refnum<vi>)
  n249 = control-ref of="BL MA 8"() -> (w412:refnum<vi>)
  n250 = control-ref of="BL MA 9"() -> (w314:refnum<vi>)
  n251 = control-ref of="PA_VacuumControl::PA_VacuumControl_PA global"() -> (w386:refnum<vi>)
  n252 = control-ref of="PA_VacuumControl::PA_VacuumControl_Telescope 1"() -> (w385:refnum<vi>)
  n253 = control-ref of="PA_VacuumControl::PA_VacuumControl_Telescope 2"() -> (w384:refnum<vi>)
  n254 = control-ref of="PA_VacuumControl::PA_VacuumControl_Telescope 3"() -> (w383:refnum<vi>)
  n255 = control-ref of="PA_VacuumControl::PA_VacuumControl_Telescope 4"() -> (w382:refnum<vi>)
  n256 = control-ref of="PA_VacuumControl::PA_VacuumControl_Bridge"() -> (w381:refnum<vi>)
  n257 = control-ref of="MA_VacuumControl::MA_VacuumControl_MA Telescope"() -> (w380:refnum<vi>)
  n258 = control-ref of="MA_VacuumControl::MA_VacuumControl_MA Telescope Prepressure"() -> (w379:refnum<vi>)
  n259 = control-ref of="MA_VacuumControl::MA_VacuumControl_Z6 Telescope BL"() -> (w315:refnum<vi>)
  n260 = control-ref of="Compressor_VacuumControl::Compressor_VacuumControl_Compressor"() -> (w288:refnum<vi>)
  n261 = control-ref of="Compressor_VacuumControl::Compressor_VacuumControl_Compressor Pre"() -> (w287:refnum<vi>)
  n262 = control-ref of="Experiment_VacuumControl::Experiment_VacuumControl_Experiment Pirani"() -> (w252:refnum<vi>)
  n263 = control-ref of="Experiment_VacuumControl::Experiment_VacuumControl_Experiment"() -> (w251:refnum<vi>)
  n264 = control-ref of="MA_VacuumControl::MA_VacuumControl_Z6 Telescope BL Prepressure"() -> (w95:refnum<vi>)
  n265 = control-ref of="MA01_O2_Beamline_MM1"() -> (w352:refnum<vi>)
  n266 = control-ref of="MA01_O2_Beamline_MM3"() -> (w351:refnum<vi>)
  n267 = control-ref of="PA_Exit_Powermeter"() -> (w358:refnum<vi>)
  n268 = control-ref of="MAS_Powermeter"() -> (w357:refnum<vi>)
  n269 = control-ref of="ns_Exit_Powermeter"() -> (w343:refnum<vi>)
  n270 = control-ref of="uOPA_Pump_Powermeter"() -> (w77:refnum<vi>)
  n271 = Build Array(w418, w417, w416, w415, w411, w414, w413, w412, w314) -> (w39:refnum<vi>[])
  n272 = control-ref of="BL PA ED 1"() -> (w362:refnum<vi>)
  n273 = control-ref of="BL PA ED 2"() -> (w361:refnum<vi>)
  n274 = control-ref of="BL Boo 1"() -> (w347:refnum<vi>)
  n275 = control-ref of="BL Boo 2"() -> (w346:refnum<vi>)
  n276 = control-ref of="BL Boo 3"() -> (w345:refnum<vi>)
  n277 = control-ref of="BL Boo 4"() -> (w344:refnum<vi>)
  n278 = control-ref of="BL Boo 5"() -> (w279:refnum<vi>)
  n279 = control-ref of="BL ns 1"() -> (w342:refnum<vi>)
  n280 = control-ref of="BL ns 2"() -> (w341:refnum<vi>)
  n281 = control-ref of="BL ns 3"() -> (w340:refnum<vi>)
  n282 = control-ref of="BL ns 4"() -> (w339:refnum<vi>)
  n283 = control-ref of="BL ns 5"() -> (w338:refnum<vi>)
  n284 = control-ref of="BL ns 6"() -> (w337:refnum<vi>)
  n285 = control-ref of="BL ns 7"() -> (w336:refnum<vi>)
  n286 = control-ref of="BL ns 8"() -> (w335:refnum<vi>)
  n287 = control-ref of="BL uOPA 4"() -> (w89:refnum<vi>)
  n288 = control-ref of="BL uOPA 0"() -> (w88:refnum<vi>)
  n289 = control-ref of="BL uOPA 6"() -> (w87:refnum<vi>)
  n290 = control-ref of="BL uOPA 9"() -> (w86:refnum<vi>)
  n291 = control-ref of="BL uOPA 2"() -> (w85:refnum<vi>)
  n292 = control-ref of="BL uOPA 7"() -> (w84:refnum<vi>)
  n293 = control-ref of="BL uOPA 1"() -> (w83:refnum<vi>)
  n294 = control-ref of="BL uOPA 3"() -> (w82:refnum<vi>)
  n295 = control-ref of="BL uOPA 5"() -> (w81:refnum<vi>)
  n296 = control-ref of="BL uOPA 8"() -> (w80:refnum<vi>)
  n297 = control-ref of="BL MA-IB 1"() -> (w378:refnum<vi>)
  n298 = control-ref of="BL MA-IB 2"() -> (w313:refnum<vi>)
  n299 = control-ref of="BL MA-IB 3"() -> (w312:refnum<vi>)
  n300 = control-ref of="BL MA-IB 4"() -> (w311:refnum<vi>)
  n301 = control-ref of="BL MA-IB 5"() -> (w310:refnum<vi>)
  n302 = control-ref of="BL MA-IB 6"() -> (w309:refnum<vi>)
  n303 = control-ref of="BL MA-IB 7"() -> (w308:refnum<vi>)
  n304 = control-ref of="BL MA-IB 8"() -> (w307:refnum<vi>)
  n305 = control-ref of="BL MA-IB 9"() -> (w306:refnum<vi>)
  n306 = control-ref of="BL MA-IB 10"() -> (w305:refnum<vi>)
  n307 = control-ref of="BL MA-IB 11"() -> (w304:refnum<vi>)
  n308 = control-ref of="BL MA-IB 12"() -> (w303:refnum<vi>)
  n309 = control-ref of="BL MA-IB 13"() -> (w302:refnum<vi>)
  n310 = control-ref of="BL MA-IB 14"() -> (w301:refnum<vi>)
  n311 = Build Array(w398, w397, w396, w395, w394, w393, w392, w391, w390, w389, w388, w387, w349) -> (w116:refnum<vi>[])
  n312 = Build Array(w358, w357, w343, w77) -> (w115:refnum<vi>[])
  n313 = Build Array(w386, w385, w384, w383, w382, w381, w380, w379, w315, w288, w287, w252, w251, w95) -> (w68:refnum<vi>[])
  n314 = Build Array(w352, w351) -> (w67:refnum<vi>[])
  n315 = Build Array(w362, w361) -> (w34:refnum<vi>[])
  n316 = Build Array(w347, w346, w345, w344, w279) -> (w32:refnum<vi>[])
  n317 = Build Array(w342, w341, w340, w339, w338, w337, w336, w335) -> (w31:refnum<vi>[])
  n318 = Build Array(w187, w186, w185, w184, w183, w182, w181, w180, w179, w174, w173, w172, w171, w170, w169, w168, w167, w166, w165, w164, w163, w162, w161, w160, w159, w158, w157, w148, w147, w136, w135, w134, w133, w132, w131, w130, w129, w128, w127, w126, w97, w76) -> (w63:refnum<vi>[])
  n319 = for {
    shift-right: [w421] -> w55
    shift-left: "error in (no error)" -> [w422]
    tunnel: w103 -> [w420] mode=indexing
    tunnel: [w419] -> w102 mode=indexing
    n320 = property class="Bool (strict)"(reference=w420, error in=w422) -> (error out=w421:errorcluster, "Label.Text"=w419:string)  [unwired: 1 out]
  }
  n321 = Build Array (concatenate)(w103, w116, w115, w114, w113, w112) -> (w65:refnum<vi>[])
  n322 = Build Array(w89, w88, w87, w86, w85, w84, w83, w82, w81, w80) -> (w28:refnum<vi>[])
  n323 = Build Array(w107, w106, w96, w4, w3) -> (w64:refnum<vi>[])
  n324 = Build Array(w377, w376, w360, w359, w350, w190, w322, w319, w318, w283, w255, w246, w208, w207, w143, w142, w141, w140) -> (w111:refnum<vi>[])
  n325 = Build Array(w334, w330, w329, w328, w327, w325, w324, w323, w300, w299, w271, w270, w254, w194) -> (w110:refnum<vi>[])
  n326 = Build Array(w280, w278) -> (w109:refnum<vi>[])
  n327 = Build Array(w267, w266) -> (w108:refnum<vi>[])
  n328 = Build Array(w189, w94, w93, w188, w124, w123, w122, w121, w120, w104, w119, w178, w177, w176, w175, w118, w117, w105) -> (w70:refnum<vi>[])
  n329 = Build Array(w124, w123, w122, w121, w120, w104, w119) -> (w125:refnum<vi>[])
  n330 = Build Array(w378, w313, w312, w311, w310, w309, w308, w307, w306, w305, w304, w303, w302, w301) -> (w36:refnum<vi>[])
  n331 = Build Array (concatenate)(w111, w110, w109, w108, w2) -> (w69:refnum<vi>[])
  n332 = control-ref of="BL Exp LB"() -> (w291:refnum<vi>)
  n333 = control-ref of="BL Exp LB 2"() -> (w290:refnum<vi>)
  n334 = control-ref of="BL Exp LB 3"() -> (w289:refnum<vi>)
  n335 = control-ref of="BL Exp LB 4"() -> (w273:refnum<vi>)
  n336 = control-ref of="BL Exp LB 5"() -> (w272:refnum<vi>)
  n337 = control-ref of="BL Exp LB 6"() -> (w193:refnum<vi>)
  n338 = control-ref of="BL Exp LB 7"() -> (w192:refnum<vi>)
  n339 = control-ref of="BL Exp LB 8"() -> (w191:refnum<vi>)
  n340 = for {
    tunnel: w125 -> [w424] mode=indexing
    n341 = property class="Pict (strict)"(reference=w424, "Caption.Visible"=FALSE) -> ()  [unwired: 1 in, 2 out]
  }
  n342 = call "PH_Interaction.get Vision IDs on same Node.vi"("Cam Instances"=w102, "i ref in"="object ref") -> ("Vision System IDs"=w99:string[], "Vision Sytem IDs found"=w57:bool, "Cams instanciated on own system"=w98:bool)  [unwired: 1 in]
  n343 = Build Array(w291, w290, w289, w273, w272, w193, w192, w191) -> (w38:refnum<vi>[])
  n344 = Index Array(array=w99) -> (element=w101:string)  [unwired: 1 in]
  n345 = control-ref of="Force Sensor Instances"() -> (w1:refnum<vi>)
  n346 = control-ref of="Switch Instances"() -> (w13:refnum<vi>)
  n347 = control-ref of="Black Box Instances"() -> (w12:refnum<vi>)
  n348 = control-ref of="6P Switch Instances"() -> (w11:refnum<vi>)
  n349 = control-ref of="Switch GUI Instances"() -> (w10:refnum<vi>)
  n350 = control-ref of="Switch and 6P Instances"() -> (w9:refnum<vi>)
  n351 = control-ref of="PHELIX_Timing_Mode"() -> (w75:refnum<vi>)
  n352 = call "PH_Interaction.set PCS System.vi"() -> ("Enum"=w286:T21)  [unwired: 1 in]
  n353 = control-ref of="Delete"() -> (w5:refnum<vi>)
  n354 = control-ref of="Ready for Shot"() -> (w66:refnum<vi>)
  n355 = Or(x=w98, y=w57) -> (x .or. y?=w16:bool)
  n356 = Select(t=w101, s=w57, f="N/A") -> (s? t:f=w62:string)
  n357 = case shown="\"Laser\"" w286 {
    tunnel: ["" "Laser" "Vision" "Pulsed Power" "Special" "Beckhoff"] -> w285
    tunnel: [TRUE TRUE TRUE TRUE FALSE FALSE] -> w284
    tunnel: [u32 0 ("Color Box") u32 16776960 ("Color Box") u32 16711935 ("Color Box") u32 65535 ("Color Box") u32 16711680 ("Color Box") u32 16448250 ("Color Box")] -> w263
    frame "PCS", Default {
    }
    frame "Laser" {
    }
    frame "Vision" {
    }
    frame "PP" {
    }
    frame "Special" {
    }
    frame "Beckhoff" {
    }
  }
  n358 = control-ref of="Laser enabled"() -> (w203:refnum<vi>)
  n359 = control-ref of="PreAmp enabled"() -> (w202:refnum<vi>)
  n360 = control-ref of="MainAmp enabled"() -> (w201:refnum<vi>)
  n361 = control-ref of="Emergency Off"() -> (w196:refnum<vi>)
  n362 = control-ref of="Shutter Exp 1"() -> (w197:refnum<vi>)
  n363 = control-ref of="Shutter Exp 2"() -> (w198:refnum<vi>)
  n364 = control-ref of="Shutter Exp 3"() -> (w199:refnum<vi>)
  n365 = control-ref of="Shutter Exp 4 (Z6)"() -> (w200:refnum<vi>)
  n366 = Bundle By Name(cluster=T18 {"Vac GUI Refs"=[], "O2 GUI Refs"=[], "Ready for Shot"=refnum, "Boolean Condition Service Subscriber GUI Refs"=[], "Vision ID on same Node"="", "Picture Condition Service Subscriber GUI Refs"=[], "6P 4Q GUI Refs"=[], "Ref Switch GUI Instances"=refnum, "Ref 6P Switch Instances"=refnum, "Ref BB Instances"=refnum, "Ref Switch Instances"=refnum, "Ref Switch and 6P State Instances"=refnum, "Boolean Status Service Subscriber GUI Refs"=[], "Picture Status Service Subscriber GUI Refs"=[], "Force Sensor Instances"=refnum, "GUI Ref Delete"=refnum} ("PH_BL_Master GUI Refs"), "Force Sensor Instances"=w1, "Ref Switch Instances"=w13, "Ref BB Instances"=w12, "Ref 6P Switch Instances"=w11, "Ref Switch GUI Instances"=w10, "Ref Switch and 6P State Instances"=w9, "Vac GUI Refs"=w68, "O2 GUI Refs"=w67, "GUI Ref Delete"=w5, "Ready for Shot"=w66, "Boolean Condition Service Subscriber GUI Refs"=w65, "Picture Condition Service Subscriber GUI Refs"=w63, "6P 4Q GUI Refs"=w64, "Boolean Status Service Subscriber GUI Refs"=w69, "Picture Status Service Subscriber GUI Refs"=w70, "Vision ID on same Node"=w62) -> (w6:T18)
  n367 = Bundle By Name(cluster=T19 {"Laser"=refnum, "PreAmp"=refnum, "MainAmp"=refnum, "Emergency Off"=refnum, "Exp 1"=refnum, "Exp 2"=refnum, "Exp 3"=refnum, "Exp 4"=refnum, "Timing Mode GUI Ref"=refnum} ("Color GUI Refs"), "Laser"=w203, "PreAmp"=w202, "MainAmp"=w201, "Emergency Off"=w196, "Exp 1"=w197, "Exp 2"=w198, "Exp 3"=w199, "Exp 4"=w200, "Timing Mode GUI Ref"=w75) -> (w7:T19)
  n368 = property on="Image Statistician" class="Bool"("Visible"=w284) -> ()  [unwired: 2 in, 2 out]
  n369 = property on="PCS System Indicator" class="Bool (strict)"("Caption.Text"=w285, "Caption.TextColor"=w263) -> ()  [unwired: 2 in, 2 out]
  n370 = control-ref of="Calibrator"() -> (w59:refnum<vi>)
  n371 = control-ref of="Igni MA 1: Heating off"() -> (w262:refnum<vi>)
  n372 = control-ref of="Igni MA 2: Heating off"() -> (w261:refnum<vi>)
  n373 = control-ref of="Igni MA 3: Heating off"() -> (w260:refnum<vi>)
  n374 = control-ref of="Igni MA 4: Heating off"() -> (w259:refnum<vi>)
  n375 = control-ref of="Igni MA 5: Heating off"() -> (w258:refnum<vi>)
  n376 = control-ref of="Igni FR: Heating off"() -> (w257:refnum<vi>)
  n377 = control-ref of="CoG"() -> (w60:refnum<vi>)
  n378 = control-ref of="PreAmp ok"() -> (w54:refnum<vi>)
  n379 = control-ref of="MainAmp ok"() -> (w53:refnum<vi>)
  n380 = control-ref of="fs Frontend ok"() -> (w52:refnum<vi>)
  n381 = control-ref of="ns Frontend ok"() -> (w51:refnum<vi>)
  n382 = control-ref of="PA ED ok"() -> (w50:refnum<vi>)
  n383 = control-ref of="In.-Box ok"() -> (w49:refnum<vi>)
  n384 = control-ref of="MAS ok"() -> (w48:refnum<vi>)
  n385 = control-ref of="Booster ok"() -> (w47:refnum<vi>)
  n386 = control-ref of="Mirrortower ok"() -> (w46:refnum<vi>)
  n387 = control-ref of="Compressor ok"() -> (w45:refnum<vi>)
  n388 = control-ref of="Experiment LB ok"() -> (w44:refnum<vi>)
  n389 = control-ref of="Laserlab ok"() -> (w43:refnum<vi>)
  n390 = control-ref of="Exp.-Shutters closed"() -> (w42:refnum<vi>)
  n391 = control-ref of="uOPA ok"() -> (w41:refnum<vi>)
  n392 = control-ref of="PHELIX_Beckhoff_Watchdog"() -> (w23:refnum<vi>)
  n393 = control-ref of="Intensity LB below Limit"() -> (w21:refnum<vi>)
  n394 = control-ref of="Intensity LL below Limit"() -> (w20:refnum<vi>)
  n395 = control-ref of="Vacuum no shotcond Comp LB"() -> (w19:refnum<vi>)
  n396 = Build Array(w60, w59) -> (w17:refnum<vi>[])
  n397 = control-ref of="Exp: Shotmode"() -> (w27:refnum<vi>)
  n398 = control-ref of="LL: Shotmode"() -> (w26:refnum<vi>)
  n399 = control-ref of="Laserbay evacuated?"() -> (w25:refnum<vi>)
  n400 = control-ref of="Laserlab evacuated?"() -> (w24:refnum<vi>)
  n401 = control-ref of="HV room locked?"() -> (w22:refnum<vi>)
  n402 = Build Array(w262, w261, w260, w259, w258, w257) -> (w18:refnum<vi>[])
  n403 = control-ref of="Tab Control"() -> ()  [unwired: 1 out]
  n404 = Bundle By Name(cluster=T17 {"Vision on this Node?"=FALSE, "Vision Knobs"=[], "GUI Refs"={"PA ok"=refnum, "MA ok"=refnum, "fs FE ok"=refnum, "ns FE ok"=refnum, "PA ED ok"=refnum, "MAS ok"=refnum, "Booster ok"=refnum, "Mirrortower ok"=refnum, "In.-Box ok"=refnum, "Compressor ok"=refnum, "Experiment LB ok"=refnum, "Experiment LL ok"=refnum, "PHELIX_Beckhoff_Watchdog"=refnum, "Shutters closed"=refnum, "uOPA ok"=refnum, "Vacuum no shotcond Comp LB"=refnum}, "PP Igni Heating GUI Refs"=[], "Refs BL PA"={"undelayed Line before Shutter"=[], "undelayed Line after Shutter"=[], "before Bypass"=[], "delayed Line before Shutter"=[], "delayed Line after Shutter"=[], "before Shutter Input"=[], "after Shutter Input"=[], "Bypass"=[], "before Shutter Exit"=[], "after Shutter Exit"=[], "to MA"=[], "to Lab"=[]}, "Refs BL MA"=[], "Refs BL MA-IB"=[], "Refs BL fs"=[], "Refs BL PA ED"=[], "Refs BL MAS"=[], "Refs BL Boo"=[], "Refs BL ns"=[], "Refs BL Mirrortower"=[], "Refs BL Compressor"=[], "Refs BL Exp LB"=[], "Refs BL LL"=[], "Refs BL uOPA"=[], "Ref Op Mode Exp LB"=refnum, "Ref Laserbay evacuated"=refnum, "Ref Op Mode Exp LL"=refnum, "Ref Laserlab evacuated"=refnum, "Ref HV room locked"=refnum, "Ref Bridge LB"=refnum, "Ref Bridge LL"=refnum} ("GUI Refs"), "GUI Refs.PA ok"=w54, "GUI Refs.MA ok"=w53, "GUI Refs.fs FE ok"=w52, "GUI Refs.ns FE ok"=w51, "GUI Refs.PA ED ok"=w50, "GUI Refs.In.-Box ok"=w49, "GUI Refs.MAS ok"=w48, "GUI Refs.Booster ok"=w47, "GUI Refs.Mirrortower ok"=w46, "GUI Refs.Compressor ok"=w45, "GUI Refs.Experiment LB ok"=w44, "GUI Refs.Experiment LL ok"=w43, "GUI Refs.Shutters closed"=w42, "GUI Refs.uOPA ok"=w41, "Refs BL PA"=w40, "Refs BL MA"=w39, "Refs BL Exp LB"=w38, "Refs BL Compressor"=w37, "Refs BL MA-IB"=w36, "Refs BL fs"=w35, "Refs BL PA ED"=w34, "Refs BL MAS"=w33, "Refs BL Boo"=w32, "Refs BL ns"=w31, "Refs BL Mirrortower"=w30, "Refs BL LL"=w29, "Refs BL uOPA"=w28, "Ref Op Mode Exp LB"=w27, "Ref Op Mode Exp LL"=w26, "Ref Laserbay evacuated"=w25, "Ref Laserlab evacuated"=w24, "GUI Refs.PHELIX_Beckhoff_Watchdog"=w23, "Ref HV room locked"=w22, "Ref Bridge LB"=w21, "Ref Bridge LL"=w20, "GUI Refs.Vacuum no shotcond Comp LB"=w19, "PP Igni Heating GUI Refs"=w18, "Vision Knobs"=w17, "Vision on this Node?"=w16) -> (w14:T17)
  n405 = control-ref of="Settings"() -> (w8:refnum<vi>)
  n406 = call "PH_Class.Register Event.vi"("i ref in"="object ref", "error in (no error)"=w55) -> ("i ref out"=w73:refnum<vi>, "Event Registration Refnum"=w61:refnum<event-registration>, "error out"=w72:errorcluster)  [unwired: 15 in]
  n407 = while {
    tunnel: w73 -> [w451]
    tunnel: [w450] -> w321
    tunnel: w72 -> [w453]
    tunnel: [w452] -> w320
    tunnel: [w448] -> w74
    tunnel: w61 -> [w447]
    tunnel: w14 -> [w446]
    tunnel: w8 -> [w445]
    tunnel: w7 -> [w444]
    tunnel: w6 -> [w443]
    stop <- w449 stop-if-true
    n408 = event shown="[7] <Event>: User Event" {
      selector: w447 -> [_ _ _ _ _ _ _ _]
      dyn-events: [_ _ _ _ _ _ _ _] -> w448
      timeout: _ -> [_ _ _ _ _ _ _ _]
      tunnel: w451 -> [w460 w465 w466 _ w489 w540 w550 w562]
      tunnel: w453 -> [w455 w464 w468 _ w495 w543 w553 w560]
      tunnel: [w459 w463 w467 _ w494 w541 w551 w564] -> w452
      tunnel: [w458 w462 w466 _ w488 w540 w552 w563] -> w450
      tunnel: ["Delete" _ _ _ _ _ _ _] -> w449
      tunnel: w446 -> [_ _ _ _ _ _ _ w558]
      tunnel: w445 -> [_ _ _ _ _ _ _ w556]
      tunnel: w444 -> [_ _ _ _ _ _ _ w555]
      tunnel: w443 -> [_ _ _ _ _ _ _ w554]
      event "Delete": Value Change {
        n409 = event-data() -> ()  [unwired: 1 in, 1 out]
        n410 = call "PH_GUI.Manager Close.vi"("i ref in"=w460, "error in"=w455) -> ("i ref out"=w456:refnum<vi>, "error out"=w454:errorcluster)  [unwired: 16 in]
        n411 = call "CSObj.open front panel.vi"("i ref in"=w456, "frontPanelOpen"=FALSE ("front panel open"), "error in (no error)"=w454) -> ("i ref out"=w458:refnum<vi>, "error out"=w459:errorcluster)  [unwired: 15 in]
      }
      event "Minimize": Value Change {
        n412 = event-data() -> ()  [unwired: 1 in, 1 out]
        n413 = call "PH_GUI.Manager Minimize.vi"("i ref in"=w465, "error in"=w464) -> ("i ref out"=w462:refnum<vi>, "error out"=w463:errorcluster)  [unwired: 16 in]
      }
      event "Remote Desktop Connection": Value Change {
        n414 = event-data() -> ()  [unwired: 1 in, 1 out]
        n415 = call "PH_Connection.select PCS Node.vi"("error in"=w468) -> ("string out"=w469:string, "error out"=w470:errorcluster)  [unwired: 17 in]
        n416 = case shown="Default" w469 {
          selector: w469 -> [_ w472]
          tunnel: w470 -> [w471 w474]
          tunnel: [w471 w473] -> w467
          frame "", "N/A" {
          }
          frame Default {
            n417 = Concatenate Strings("mstsc " ("command line"), w472) -> (w476:string)
            n418 = call <vilib>:"System Exec.vi"("wait until completion? (T)"=FALSE, "error in (no error)"=w474, "command line"=w476) -> ("error out"=w473:errorcluster)  [unwired: 5 in, 3 out]
          }
        }
      }
      event "Hop 1", "Hop 2", "Hop 3", "Hop 4", "Hop 5", "Hop 6", "Hop 7", "Hop 8", "Hop 9", "Hop 10", "Hop 11", "Hop 12", "Hop 13", "Hop 14", "Hop 15", "Hop 16", "Hop 17", "Hop 18", "Hop 19", "Hop 20", "Hop 21", "Hop 22", "Hop 23", "Hop 24": Value Change {
        n419 = event-data() -> ("CtlRef"=w482:refnum<vi>)  [unwired: 1 in]
        n420 = property on="Tab Control" class="TabCtl (strict)"() -> ("Pages"=w481:refnum<vi>[])  [unwired: 2 in, 2 out]
        n421 = for {
          tunnel: [w485] -> w480 mode=indexing
          tunnel: w481 -> [w484] mode=indexing
          n422 = property class="Page"(reference=w484) -> ("Page Label"=w485:string)  [unwired: 1 in, 2 out]
        }
        n423 = property class="Bool"(reference=w482) -> ("Boolean Text.Text"=w479:string)  [unwired: 1 in, 2 out]
        n424 = Search 1D Array(1D array=w480, element=w479) -> (index of element=w478:i32)  [unwired: 1 in]
        n425 = case shown="Default" w478 {
          selector: w478 -> [_ w483]
          frame -1 {
          }
          frame Default {
            n426 = property on="Tab Control" class="TabCtl (strict)"("Value"=w483) -> ()  [unwired: 2 in, 2 out]
          }
        }
      }
      event "Image Statistician", "Calibrator", "PCS Main", "CoG", "Z6 Main", "Z6 Beamline": Value Change {
        n427 = event-data() -> ("CtlRef"=w493:refnum<vi>)  [unwired: 1 in]
        n428 = property class="Bool"(reference=w493, error in=w495) -> (error out=w487:errorcluster, "Label.Text"=w492:string)  [unwired: 1 out]
        n429 = case shown="\"CoG\"" w492 {
          tunnel: [T22."None" ("Instance to create or open") T22."PCS Main" ("Instance to create or open") T22."Z6 Main" ("Instance to create or open") T22."Z6 Beamline" ("Instance to create or open") T22."Image Statistician" ("Instance to create or open") T22."Image Center of Gravity" ("Instance to create or open") T22."Image Calibrator" ("Instance to create or open")] -> w491
          tunnel: ["N/A" ("Vision ID on same Node") "N/A" "N/A" "N/A" "N/A" w516 w523] -> w490
          tunnel: w487 -> [w497 w500 w504 w508 w512 w519 w528]
          tunnel: w489 -> [w498 w501 w505 w509 w513 w520 w527]
          tunnel: [w498 w501 w505 w509 w513 w518 w526] -> w488
          tunnel: [w497 w500 w504 w508 w512 w517 w525] -> w486
          frame Default {
          }
          frame "PCS Main" {
          }
          frame "Z6 Main" {
          }
          frame "Z6 Beamline" {
          }
          frame "Image Statistician" {
          }
          frame "CoG" {
            n430 = call "PH_BL-Master.get i attribute.vi"("i ref in"=w520, "error in (no error)"=w519) -> ("i ref out"=w518:refnum<vi>, "i attribute"=w521:T23, "error out"=w517:errorcluster)  [unwired: 15 in]
            n431 = Unbundle By Name(w521) -> ("Vision ID on same Node"=w516:string)
          }
          frame "Calibrator" {
            n432 = call "PH_BL-Master.get i attribute.vi"("i ref in"=w527, "error in (no error)"=w528) -> ("i ref out"=w526:refnum<vi>, "i attribute"=w524:T23, "error out"=w525:errorcluster)  [unwired: 15 in]
            n433 = Unbundle By Name(w524) -> ("Vision ID on same Node"=w523:string)
          }
        }
        n434 = call "PH_Interaction.Open or Create PCS Instances.vi"("System ID (N/A)"=w490, "Instance to create or open"=w491, "error IO"=w486) -> ("error out"=w494:errorcluster)  [unwired: 16 in]
      }
      event "\"D:\\PCS\\Remote Access\\ns.rdp\"", "\"D:\\PCS\\Remote Access\\fs.rdp\"", "\"D:\\PCS\\Remote Access\\PA-Input.rdp\"", "\"D:\\PCS\\Remote Access\\PA-Exit.rdp\"", "\"D:\\PCS\\Remote Access\\MA.rdp\"", "\"D:\\PCS\\Remote Access\\MA.rdp\" 2", "\"D:\\PCS\\Remote Access\\MAS.rdp\"", "\"D:\\PCS\\Remote Access\\COS.rdp\"", "\"D:\\PCS\\Remote Access\\Experiment.rdp\"", "\"D:\\PCS\\Remote Access\\Laserlabor.rdp\"", "\"D:\\PCS\\Remote Access\\uOPA.rdp\"": Value Change {
        n435 = event-data() -> ("CtlRef"=w544:refnum<vi>)  [unwired: 1 in]
        n436 = property class="Bool"(reference=w544, error in=w543) -> (error out=w530:errorcluster, "Label.Text"=w531:string)  [unwired: 1 out]
        n437 = Match Pattern(string=w531, regular expression=" 2") -> (before substring=w532:string, offset past match=w536:i32)  [unwired: 1 in, 2 out]
        n438 = Equal?(x=w536, y=-1) -> (x = y?=w534:bool)
        n439 = Select(t=w531, s=w534, f=w532) -> (s? t:f=w533:string)
        n440 = Concatenate Strings("mstsc " ("command line"), w533) -> (w539:string)
        n441 = call <vilib>:"System Exec.vi"("wait until completion? (T)"=FALSE, "error in (no error)"=w530, "command line"=w539) -> ("error out"=w541:errorcluster)  [unwired: 5 in, 3 out]
      }
      event Value Change {
        n442 = event-data() -> ("CtlRef"=w546:refnum<vi>, "OldVal"=w545:T16, "NewVal"=w548:T16)  [unwired: 1 in]
        n443 = property class="Clust (strict)"(reference=w546, error in=w553, "Value"=w545) -> (error out=w547:errorcluster)  [unwired: 1 out]
        n444 = call "CSSystemLib.ref2name.vi"("obj refnum"=w550) -> ("name"=w549:string)
        n445 = call "PH_Beamline_Chief.Event Call Set Settings.vi"("VI in"=w550, "Instance"=w549, "Settings"=w548, "error in (no error)"=w547) -> ("VI out"=w552:refnum<vi>, "error out"=w551:errorcluster)  [unwired: 14 in]
      }
      event User Event {
        n446 = event-data() -> ("Class"=w557:string)  [unwired: 1 in]
        n447 = case shown="Default" w557 {
          selector: w557 -> [_ w580]
          tunnel: w562 -> [w576 w584]
          tunnel: [w572 w583] -> w561
          tunnel: w560 -> [w575 w582]
          tunnel: [w568 w581] -> w559
          tunnel: w558 -> [_ w577]
          tunnel: w556 -> [w567 _]
          tunnel: w555 -> [_ w579]
          tunnel: w554 -> [_ w578]
          frame "PH_Beamline_Chief" {
            n448 = call "PH_Beamline_Chief.get data to modify.vi"("i ref in"=w576, "ms timeout (10000)"=-1, "error in (no error)"=w575) -> ("i ref out"=w574:refnum<vi>, "i attribute"=w569:T27, "error out"=w573:errorcluster)  [unwired: 13 in, 1 out]
            n449 = Bundle By Name(cluster=w569, "Settings.GUI Ref"=w567) -> (w566:T27)
            n450 = call "PH_Beamline_Chief.set modified data.vi"("i ref in"=w574, "i attribute"=w566, "error in (no error)"=w573) -> ("i ref out"=w572:refnum<vi>, "error out"=w571:errorcluster)  [unwired: 15 in]
            n451 = Unbundle By Name(w566) -> ("Settings.Wanted"=w565:T16)
            n452 = property class="Clust (strict)"(reference=w567, error in=w571, "Value"=w565) -> (error out=w568:errorcluster)  [unwired: 1 out]
          }
          frame Default {
            n453 = call "PH_Beamline.set GUI Refs.vi"("i ref in"=w584, "Class"=w580, "PH Beamline GUI Refs"=w577, "PH_BL-Master GUI Refs"=w578, "System Information GUI Refs"=w579, "error in (no error)"=w582) -> ("i ref out"=w583:refnum<vi>, "error out"=w581:errorcluster)  [unwired: 12 in]
          }
        }
        n454 = call "PH_Class.set GUI Refs stored Occurence.vi"("i ref in"=w561, "error in (no error)"=w559) -> ("i ref out"=w563:refnum<vi>, "error out"=w564:errorcluster)  [unwired: 16 in]
      }
    }
  }
  "error out" <- w320
  n455 = property on="PA_Bypass_In" class="Pict (strict)"("Disabled"=w253) -> ()  [unwired: 2 in, 2 out]
  n456 = property on="PA_Bypass_Out" class="Pict (strict)"("Disabled"=w253) -> ()  [unwired: 2 in, 2 out]
  n457 = property on="PA_PC_WP_BB" class="Bool (strict)"("Disabled"=w253) -> ()  [unwired: 2 in, 2 out]
  n458 = property on="Shutter_Exp1" class="Bool (strict)"("Disabled"=w253) -> ()  [unwired: 2 in, 2 out]
  n459 = property on="Shutter_Exp2" class="Bool (strict)"("Disabled"=w253) -> ()  [unwired: 2 in, 2 out]
  n460 = property on="Shutter_Exp3" class="Bool (strict)"("Disabled"=w253) -> ()  [unwired: 2 in, 2 out]
  n461 = property on="Shutter_Exp4" class="Bool (strict)"("Disabled"=w253) -> ()  [unwired: 2 in, 2 out]
  n462 = property on="PA_PC_WP_2_BB" class="Bool (strict)"("Disabled"=w253) -> ()  [unwired: 2 in, 2 out]
  n463 = Unregister For Events(event registration refnum=w74) -> ()  [unwired: 1 in, 1 out]
  n464 = call "PH_Interaction.Super Destroy Me.vi"("i ref out"=w321) -> ()
